vi "Steuerprogramm_ECD.vi"() -> ()   [LabVIEW 2017]
uses:
  <vilib>/FPGAPlugInAG/cRIO-9035/niLvFpga_Close_cRIO-9035.vi
  <vilib>/rvi/errors/niLvFpgaAdjustHostInterfaceError.vi
  <vilib>/Utility/error.llb/Error Cluster From Error Code.vi
  GVZeitenZyklen.vi
  GVHorstSP.vi
  gvbooleschRT.vi
  GVMethodenwechsel.vi
  GVaktuelleTDMS.vi
  GVChroms.vi
  GVMWHorst.vi
  GVVentilposition.vi
  GVMetavariablen.vi
  GVHK1Hz.vi
  GVZwangs.vi
  GVZwangsMPV.vi
  GVTrapsMachs.vi
  GVECDs.vi
  GVAIs.vi
  GVHeizenLH.vi
  GVProbenvol.vi
  <vilib>/rvi/interface/nirviCloseFPGA/nirviCloseFPGA.xnode
  FPGA Bitfiles/HAGAR-VECD_FPGATarget_FPGA-ProgrammECD_WS++LmW9gGg.lvbitx
  FPGA-Programm_ECD.vi
  <vilib>/rvi/interface/nirviReadWriteControl/nirviReadWriteControl.xnode
  <vilib>/rvi/interface/nirviMethod/nirviMethod.xnode
  <vilib>/rvi/errors/niLvFpgaMergeErrorWithErrorCode.vi
  <vilib>/FPGAPlugInAG/cRIO-9035/niLvFpga_WriteFifo_cRIO-9035.vi
  NiFpgaLv.dll
panel:
  in  "Methode speichern":bool
  out "ZyklusNummernGesamt":i32[](array[numeric])
  in  "veränderte Methode benutzen":bool
  in  "Methode verändern":bool
  out "ZyklusNummern":i32[](array[numeric])
  out "Big Ben, Methodenzeit, Zykluszeit0, Zykluszeit1, Zykluszeit2A, Zykluszeit2B":i32[](array[numeric])
  in  "global stop RT":bool
  in  "Methode":i32(ring) items=["Bedingsmethode", "Startmethode", "Meßmodus", "Shut-up-Methode", "Test", "HAG2 1/2", "Startmethode", "HAG2 1/2 Aufwärmen", "LicorDruckProfil1", "LicorDruckProfil2", "LicorDruckProfil0", "LicorDruckProfil3", "Kalibration-Meßmodus", "Kalibration-Meßmodus-II", "Kalibration-MesmodusIII", "Kalibration-Messmodus-IV", "Kalibration-ECD", "", "Kalibration-ECD-Blank"]
  in  "Registerkarte":T1(tab)
  out "SHOK?":bool[](array[boolean])
  out "schnelle Heizungen":string[](array[string])
  out "schnelle Heizungen":dbl[](array[numeric])
  out "HorstOK?":bool[](array[boolean])
  out "AIs3OK?":bool[](array[boolean])
  out "AIs1OK?":bool[](array[boolean])
  out "AIs1":dbl[](array[numeric])
  out "AIs1":string[](array[string])
  out "AIs2":string[](array[string])
  out "AIs3":string[](array[string])
  out "AIs2":dbl[](array[numeric])
  out "AIs3":dbl[](array[numeric])
  out "Metavariablen":string[](array[string])
  out "Metavariablen":dbl[](array[numeric])
  out "MWHorst":dbl[](array[numeric])
  out "HorstRegler":string[](array[string])
  out "AIs2OK?":bool[](array[boolean])
  out "Ventilposition":i32=1 min=1 max=6 step=1
  out "MVOK?":bool[](array[boolean])
  in  "LH-Gruppe":bool[](array[boolean])=[FALSE, FALSE, FALSE, FALSE, FALSE, FALSE, FALSE, FALSE, FALSE, FALSE, FALSE, FALSE]
  out "LangsameHeizungen":string[](array[string])
  out "Housekeeping1":cluster{dbl[], dbl[]}(graph)
  in  "Zeitachse1":i32(ring)=1 items=["Zykluszeit [s] Mod0", "Zykluszeit [s] Mod1", "Zykluszeit [s] Mod2A", "Zykluszeit [s] Mod2B"]
  in  "dargestellte Größe 1":i32(ring)=1 items=["T1-Spare1", "T1-Spare2", "T1-StirlingKühlkopf [°C]", "T1-PreCol1 [°C]", "T1-PreCol2 [°C]", "T1-MainCol1a [°C]", "T1-MainCol1b [°C]", "T1-MainCol2a [°C]", "T1-MainCol2b [°C]", "T1-BronkhorstUntena [°C]", "T1-BronkhorstUntenb [°C]", "T1-BronkhorstObena [°C]", "T1-BronkhorstObenb [°C]", "T1-2Pos1B [°C]", "T1-Spare9", "T1-2Pos1A [°C]", "T1-Spare10", "T1-TurboPump [°C]", "T1-StirlingPlatine [°C]", "T1-Spare5", "T1-Spare6", "T1-Spare7", "T1-Inlet [°C]", "F1-MFM-Spare", "F1-MFM0D [mL]", "P1-HeliumHP [bara]", "P1-HeliumLP [bara]", "P1-PumpVordruck [mbara]", "TurboSpeed", "I1-MS-AC [A]", "I1-Trap1 [A]", "I1-Trap2 [A]", "T2-ECD1a", "T2-ECD1b", "T2-ECD2a", "T2-ECD2b", "T2-Col1a", "T2-Col1b", "T2-Col2a", "T2-Col2b", "T2-Spare1", "T2-Spare2", "T2-Spare3", "T2-Spare4", "T2-Spare5", "T2-Spare6", "T2-Spare7", "F2-MFM2A", "F2-MFM2B", "F2-MFM2C", "P2-N2O_HP", "P2-N2O_LP", "P2-CO2_HP", "P2-CO2_LP", "AI-Spare1", "FL-MFM1000mL", "AI-Spare3", "AI-Spare4", "StirlingAlarm", "StirlingEmerg.", "AI-Spare7", "AI-Spare8", "AI-Spare9", "FL-MFM30mL", "T0-DC/DC5", "I0-24V_M0", "I0-48V_M1", "I0-24V_M1", "I0-28V_M2", "T0-Spare3", "T0-Spare2", "T0-Spare4", "T0-DC/DC7", "I0-20V_Laptop", "I0-28V_M1", "I0-24V_M2", "I0-12V_Licor", "T0-Spare1", "T0-Drier", "T0-Spare5", "F0-MFM0A [L]", "TL-Licor_a", "P0-Span-HP", "P0-spare1", "P0-Stickstoff-LP", "P0-Helium-LP", "P0-Cal-HP", "P0-P9Tavco[bar]", "F0-MFM0B [L]", "TL-Licor_b", "P0-Span-LP", "P0-spare2", "P0-Stickstoff-HP", "P0-Helium-HP", "P0-Cal-LP", "F0-MFM3", "TemperaturTrap1[°C]", "TemperaturTrap2[°C]", "TemperaturPreMach1[°C]", "TemperaturPreMach2[°C]", "TemperaturMainMach1[°C]", "TemperaturMainMach2[°C]", "PrC0 [bara]", "PrC0-Licor [bara]", "PrC1-Säule1 [bara]", "PrC1-Säule2 [bara]", "MFC1-Sample [ml/min]", "PrC1-BackFlush1 [bara]", "PrC1-BackFlush2 [bara]", "MFC1-Reaktant [l/min]", "MFC2A[ml/min]", "MFC2B[ml/min]", "MFC2C[ul/min]", "PrC2A[bara]", "MFC2D[ml/min]", "MFC2E[ml/min]", "PrC2B[bara]"]
  out "Housekeeping2":cluster{dbl[], dbl[]}(graph)
  in  "Zeitachse2":i32(ring)=1 items=["Zykluszeit [s] Mod0", "Zykluszeit [s] Mod1", "Zykluszeit [s] Mod2A", "Zykluszeit [s] Mod2B"]
  in  "dargestellte Größe 2":i32(ring)=1 items=["T1-Spare1", "T1-Spare2", "T1-StirlingKühlkopf [°C]", "T1-PreCol1 [°C]", "T1-PreCol2 [°C]", "T1-MainCol1a [°C]", "T1-MainCol1b [°C]", "T1-MainCol2a [°C]", "T1-MainCol2b [°C]", "T1-BronkhorstUntena [°C]", "T1-BronkhorstUntenb [°C]", "T1-BronkhorstObena [°C]", "T1-BronkhorstObenb [°C]", "T1-2Pos1B [°C]", "T1-Spare9", "T1-2Pos1A [°C]", "T1-Spare10", "T1-TurboPump [°C]", "T1-StirlingPlatine [°C]", "T1-Spare5", "T1-Spare6", "T1-Spare7", "T1-Inlet [°C]", "F1-MFM-Spare", "F1-MFM0D [mL]", "P1-HeliumHP [bara]", "P1-HeliumLP [bara]", "P1-PumpVordruck [mbara]", "TurboSpeed", "I1-MS-AC [A]", "I1-Trap1 [A]", "I1-Trap2 [A]", "T2-ECD1a", "T2-ECD1b", "T2-ECD2a", "T2-ECD2b", "T2-Col1a", "T2-Col1b", "T2-Col2a", "T2-Col2b", "T2-Spare1", "T2-Spare2", "T2-Spare3", "T2-Spare4", "T2-Spare5", "T2-Spare6", "T2-Spare7", "F2-MFM2A", "F2-MFM2B", "F2-MFM2C", "P2-N2O_HP", "P2-N2O_LP", "P2-CO2_HP", "P2-CO2_LP", "AI-Spare1", "FL-MFM1000mL", "AI-Spare3", "AI-Spare4", "StirlingAlarm", "StirlingEmerg.", "AI-Spare7", "AI-Spare8", "AI-Spare9", "FL-MFM30mL", "T0-DC/DC5", "I0-24V_M0", "I0-48V_M1", "I0-24V_M1", "I0-28V_M2", "T0-Spare3", "T0-Spare2", "T0-Spare4", "T0-DC/DC7", "I0-20V_Laptop", "I0-28V_M1", "I0-24V_M2", "I0-12V_Licor", "T0-Spare1", "T0-Drier", "T0-Spare5", "F0-MFM0A [L]", "TL-Licor_a", "P0-Span-HP", "P0-spare1", "P0-Stickstoff-LP", "P0-Helium-LP", "P0-Cal-HP", "P0-P9Tavco[bar]", "F0-MFM0B [L]", "TL-Licor_b", "P0-Span-LP", "P0-spare2", "P0-Stickstoff-HP", "P0-Helium-HP", "P0-Cal-LP", "F0-MFM3", "TemperaturTrap1[°C]", "TemperaturTrap2[°C]", "TemperaturPreMach1[°C]", "TemperaturPreMach2[°C]", "TemperaturMainMach1[°C]", "TemperaturMainMach2[°C]", "PrC0 [bara]", "PrC0-Licor [bara]", "PrC1-Säule1 [bara]", "PrC1-Säule2 [bara]", "MFC1-Sample [ml/min]", "PrC1-BackFlush1 [bara]", "PrC1-BackFlush2 [bara]", "MFC1-Reaktant [l/min]", "MFC2A[ml/min]", "MFC2B[ml/min]", "MFC2C[ul/min]", "PrC2A[bara]", "MFC2D[ml/min]", "MFC2E[ml/min]", "PrC2B[bara]"]
  out "Detektor 2":cluster{dbl[], dbl[]}[](graph)
  in  "Detektor":i32(ring) items=["ECD1", "ECD2"]
  in  "HK1YMin":dbl
  in  "HK1YMax":dbl=100.0
  in  "HK2YMin":dbl
  in  "HK2YMax":dbl=100.0
  in  "DetYMin":dbl
  in  "DetYMax":dbl=100.0
  in  "NeuerRefstrom":bool
  in  "RefStromECD1":i16 min=0 max=2500 step=1
  in  "RefStromECD2":i16 min=0 max=2500 step=1
  out "schnelleAnzeige":cluster{dbl[], dbl[]}(graph)
  in  "TafelWischen!":bool
  in  "dargestellte Größe 3":i32(ring)=1 items=["TemperaturTrap1[°C]", "TemperaturTrap2[°C]", "TemperaturPreMach1[°C]", "TemperaturPreMach2[°C]", "TemperaturMainMach1[°C]", "TemperaturMainMach2[°C]", "PrC0 [bara]", "PrC0-Licor [bara]", "PrC1-Säule1 [bara]", "PrC1-Säule2 [bara]", "MFC1-Sample [ml/min]", "PrC1-BackFlush1 [bara]", "PrC1-BackFlush2 [bara]", "MFC1-Reaktant [l/min]", "MFC2A[ml/min]", "MFC2B[ml/min]", "MFC2C[ul/min]", "PrC2A[bara]", "MFC2D[ml/min]", "MFC2E[ml/min]", "PrC2B[bara]"]
  in  "An/Aus":bool
  out "TDMSwriteECD":errorcluster
  out "AIsFIFOread":errorcluster
  out "MWTrapsMachs":errorcluster
  out "TDMSwriteHK":errorcluster
  out "TDMScloseHK":errorcluster
  out "TDMSopenHK":errorcluster
  out "TDMScloseECD2":errorcluster
  out "TDMSopenECD2":errorcluster
  out "TDMScloseECD1":errorcluster
  out "TDMSopenECD1":errorcluster
  out "FIFOwriteRS485":errorcluster
  out "SerielleKomm.":errorcluster
  out "LH":errorcluster
  out "Zyklus":errorcluster
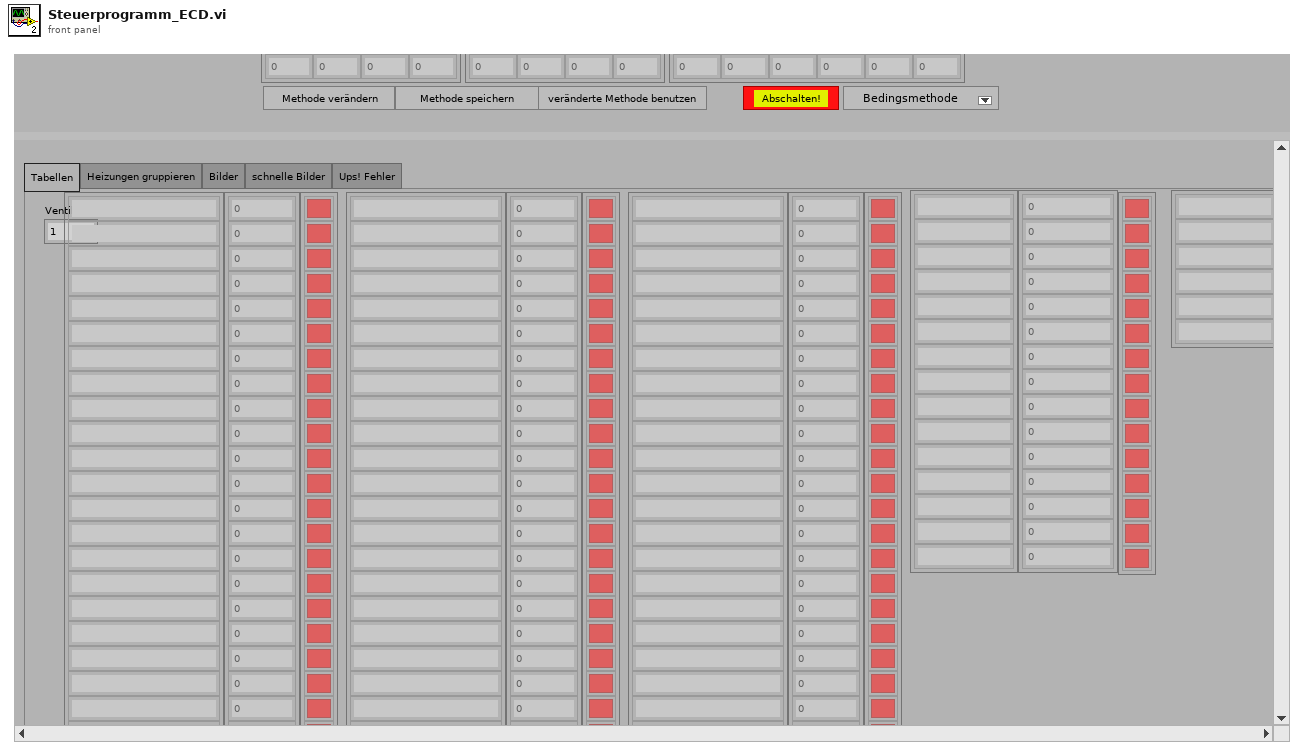
[diagram p1: front panel]
types:
  T1 = enum32{"Tabellen", "Heizungen gruppieren", "Bilder", "schnelle Bilder", "Ups! Fehler"}
  T2 = cluster{"DIOsMod0Nr":i32[], "DIOsMod1Nr":i32[], "DIOsMod2ANr":i32[], "DIOsMod2BNr":i32[], "AIsLH":i32[], "AnzahlRegler/Modul":i32[], "Regler für den Probenfluß":i32, "SPvorgebenMod0":string[], "SPvorgebenMod1":string[], "SPvorgebenMod2A":string[], "SPvorgebenMod2B":string[], "MWAntwortMod0":string[], "MWAntwortMod1":string[], "MWAntwortMod2A":string[], "MWAntwortMod2B":string[], "FaktorMod0":dbl[], "FaktorMod1":dbl[], "FaktorMod2A":dbl[], "FaktorMod2B":dbl[], "MWabfragenMod0":string[], "MWabfragenMod1":string[], "MWabfragenMod2A":string[], "MWabfragenMod2B":string[], "Modul1/AI koeff":dbl[][], "Modul2/AI koeff":dbl[][], "Modul3/AI koeff":dbl[][], "Traps/MachsKoeff T(R)":dbl[][], "Modul1/AIsNamen":string[], "Modul2/AIsNamen":string[], "Modul3/AIsNamen":string[], "DIOsMod0Name":string[], "DIOsMod1Name":string[], "DIOsMod2AName":string[], "DIOsMod2BName":string[], "ReglerNameMod0":string[], "ReglerNameMod1":string[], "ReglerNameMod2A":string[], "ReglerNameMod2B":string[], "Startmethode":i32, "Dateiordner Housekeeping":path, "Dateiname Housekeeping":string, "DateiordnerECD1":path, "DateinameECD1":string, "DateiordnerECD2":path, "DateinameECD2":string, "LangsameHeizungen":string[], "ModuleLH":i32[], "Metavariablen":string[], "Modul1/AI sicherer Bereich":dbl[][], "Modul2/AI sicherer Bereich":dbl[][], "Modul3/AI sicherer Bereich":dbl[][], "Traps/Machs sicherer Bereich":dbl[][], "ReglerMod0 sicherer Bereich":dbl[][], "ReglerMod1 sicherer Bereich":dbl[][], "ReglerMod2A sicherer Bereich":dbl[][], "ReglerMod2B sicherer Bereich":dbl[][], "Metavariablen grüner Bereich":dbl[][], "Traps/MachsKoeff R(U)":dbl[][], "LHGruppe":bool[]}
  T3 = cluster{"Zykluslängen [s]":dbl[], "ZeitpktDIOsMod0":dbl[], "ZeitpktDIOsMod1":dbl[], "ZeitpktDIOsMod2A":dbl[], "ZeitpktDIOsMod2B":dbl[], "DIOsSPMod0":bool[][], "DIOsSPMod1":bool[][], "DIOsSPMod2A":bool[][], "DIOsSPMod2B":bool[][], "Mod0HorstZeitpkt":dbl[], "Mod1HorstZeitpkt":dbl[], "Mod2AHorstZeitpkt":dbl[], "Mod2BHorstZeitpkt":dbl[], "HorstSPMod0":dbl[][], "HorstSPMod1":dbl[][], "HorstSPMod2A":dbl[][], "HorstSPMod2B":dbl[][], "LHSetpoints":dbl[], "LHHeizen?":bool[], "ZPktFPGABoolesch":dbl[], "FPGABoolesch":bool[][], "ZeitpktFPGAPID":dbl[], "FPGAPID":cluster{"d0":fxp<+/-,18,18>, "d1":fxp<+/-,21,21>}[][], "ZeitpktFPGAFixp":dbl[], dbl[][], "t_PreMach1":dbl[], "T_PreMach1":dbl[], "t_PreMach2":dbl[], "T_PreMach2":dbl[], "PIDs für \"träge\" Heizungen":cluster{"proportional gain (Kc)":dbl, "integral time (Ti, min)":dbl, "derivative time (Td, min)":dbl}[], "Zwangsbedingungen":dbl[][], "Dateien fürs MS schicken?":bool, "ZeitpunkteMPV":dbl[], "SPMPV":i32[], "ZeitpktMS-1":dbl, "ZeitpktMS-2":dbl, "Int.Start1":dbl, "Int.Stop1":dbl, "Int.Start2":dbl, "Int.Stop2":dbl, "Methodenname":string, "t_MainMach1":dbl[], "T_MainMach1":dbl[], "t_MainMach2":dbl[], "T_MainMach2":dbl[]}[]
  T4 = enum16{"open", "replace", "create", "open or create", "replace or create", "replace or create with confirmation"}
  T5 = cluster{"Zyklus1":i32, "Zeitachse1":i32, "dargestellte Größe 1":i32, "Zyklus2":i32, "Zeitachse2":i32, "dargestellte Größe 2":i32}
  T6 = cluster{"DIOsMod0Name":string[], "DIOsMod1Name":string[], "DIOsMod2AName":string[], "DIOsMod2BName":string[], "ReglerNameMod0":string[], "ReglerNameMod1":string[], "ReglerNameMod2A":string[], "ReglerNameMod2B":string[], "LangsameHeizungen":string[]}
  T7 = cluster{"Zykluslängen [s]":dbl[], "ZeitpktDIOsMod0":dbl[], "ZeitpktDIOsMod1":dbl[], "ZeitpktDIOsMod2A":dbl[], "ZeitpktDIOsMod2B":dbl[], "DIOsSPMod0":bool[][], "DIOsSPMod1":bool[][], "DIOsSPMod2A":bool[][], "DIOsSPMod2B":bool[][], "Mod0HorstZeitpkt":dbl[], "Mod1HorstZeitpkt":dbl[], "Mod2AHorstZeitpkt":dbl[], "Mod2BHorstZeitpkt":dbl[], "HorstSPMod0":dbl[][], "HorstSPMod1":dbl[][], "HorstSPMod2A":dbl[][], "HorstSPMod2B":dbl[][], "LHSetpoints":dbl[], "LHHeizen?":bool[], "ZPktFPGABoolesch":dbl[], "FPGABoolesch":bool[][], "ZeitpktFPGAPID":dbl[], "FPGAPID":cluster{"d0":fxp<+/-,18,18>, "d1":fxp<+/-,21,21>}[][], "ZeitpktFPGAFixp":dbl[], dbl[][], "t_PreMach1":dbl[], "T_PreMach1":dbl[], "t_PreMach2":dbl[], "T_PreMach2":dbl[], "PIDs für \"träge\" Heizungen":cluster{"proportional gain (Kc)":dbl, "integral time (Ti, min)":dbl, "derivative time (Td, min)":dbl}[], "Zwangsbedingungen":dbl[][], "Dateien fürs MS schicken?":bool, "ZeitpunkteMPV":dbl[], "SPMPV":i32[], "ZeitpktMS-1":dbl, "ZeitpktMS-2":dbl, "Int.Start1":dbl, "Int.Stop1":dbl, "Int.Start2":dbl, "Int.Stop2":dbl, "Methodenname":string, "t_MainMach1":dbl[], "T_MainMach1":dbl[], "t_MainMach2":dbl[], "T_MainMach2":dbl[]}
  T8 = cluster{"Modul1/AI sicherer Bereich":dbl[][], "Modul2/AI sicherer Bereich":dbl[][], "Modul3/AI sicherer Bereich":dbl[][], "Traps/Machs sicherer Bereich":dbl[][], dbl[][], "Metavariablen grüner Bereich":dbl[][]}
  T9 = cluster{"created path":path, "created path":path, "created path":path, "Dateiname Housekeeping":string, "DateinameECD1":string, "DateinameECD2":string, "tdms0":refnum<k34>, "tdms1":refnum<k34>, "tdms0":refnum<k34>, "tdms1":refnum<k34>, "tdms0":refnum<k34>, "tdms1":refnum<k34>}
  T10 = cluster{"d0":fxp<+/-,18,18>, "d1":fxp<+/-,21,21>}[][]
  T11 = cluster{"proportional gain (Kc)":dbl, "integral time (Ti, min)":dbl, "derivative time (Td, min)":dbl}[]
  T12 = cluster{cluster{"ZeitpktDIOsMod2B":dbl[]}[], cluster{"DIOsSPMod2B":bool[][]}[], cluster{"Mod2BHorstZeitpkt":dbl[]}[], cluster{"HorstSPMod2B":dbl[][]}[], "LHHeizen?":bool[], "ZPktFPGABoolesch":dbl[], "FPGABoolesch":bool[][], "ZeitpktFPGAPID":dbl[], "FPGAPID":cluster{"d0":fxp<+/-,18,18>, "d1":fxp<+/-,21,21>}[][], "ZeitpktFPGAFixp":dbl[], dbl[][], "t_PreMach1":dbl[], "T_PreMach1":dbl[], "t_PreMach2":dbl[], "T_PreMach2":dbl[], "ZeitpunkteMPV":dbl[], "SPMPV":i32[], "t_MainMach1":dbl[], "T_MainMach1":dbl[], "t_MainMach2":dbl[], "T_MainMach2":dbl[]}
  T13 = cluster{"Zykluslängen [s]":dbl[], "ZeitpktDIOsMod0":dbl[], "ZeitpktDIOsMod1":dbl[], "ZeitpktDIOsMod2A":dbl[], "ZeitpktDIOsMod2B":dbl[], "DIOsSPMod0":bool[][], "DIOsSPMod1":bool[][], "DIOsSPMod2A":bool[][], "DIOsSPMod2B":bool[][], "Mod0HorstZeitpkt":dbl[], "Mod1HorstZeitpkt":dbl[], "Mod2AHorstZeitpkt":dbl[], "Mod2BHorstZeitpkt":dbl[], "HorstSPMod0":dbl[][], "HorstSPMod1":dbl[][], "HorstSPMod2A":dbl[][], "HorstSPMod2B":dbl[][], "LangsameHeizungenSP":dbl[], "LHHeizen?":bool[], "ZPktFPGABoolesch":dbl[], "FPGABoolesch":bool[][], "ZeitpktFPGAPID":dbl[], "FPGAPID":cluster{"d0":fxp<+/-,18,18>, "d1":fxp<+/-,21,21>}[][], "ZeitpktFPGAFixp":dbl[], "FPGAFixp":dbl[][], "t_PreMach1":dbl[], "T_PreMach1":dbl[], "t_PreMach2":dbl[], "T_PreMach2":dbl[], "PIDs für \"träge\" Heizungen":cluster{"proportional gain (Kc)":dbl, "integral time (Ti, min)":dbl, "derivative time (Td, min)":dbl}[], "Zwangsbedingungen":dbl[][], "MS-Daten?":bool, "ZeitpunkteMPV":dbl[], "SetpointMPV":i32[], "ZeitpktMS-1":dbl, "ZeitpktMS-2":dbl, "Int.Start1":dbl, "Int.Stop1":dbl, "Int.Start2":dbl, "Int.Stop2":dbl, "Methodenname":string, "t_MainMach1":dbl[], "T_MainMach1":dbl[], "t_MainMach2":dbl[], "T_MainMach2":dbl[]}
  T14 = cluster{"ZyklusNummern":i32[], "ZeilennummernDIOs":i32[], "ZwangsDIO?":cluster{bool[]}[], "ZeilennummernHorst":i32[], "ZwangsHorst?":cluster{bool[]}[], "ZeileFPGABoolesch":i32, "ZwangsFPGABoolesch?":bool[], "ZeileFPGAPID":i32, "ZeileFPGAFixp":i32, "ZeilePreMach1":i32, "ZeilePreMach2":i32, "ZeilennummerMPV":i32, "ZeileMainMach1":i32, "ZeileMainMach2":i32, "ZwangsMPV?":bool}
  T15 = cluster{"ZyklusNummern":i32[], i32[], "ZwangsDIO?":cluster{bool[]}[], i32[], "ZwangsHorst?":cluster{bool[]}[], i32, "ZwangsFPGABoolesch?":bool[], i32, i32, "ZeileMach":i32, "ZeileMach":i32, i32, "ZeileMach":i32, "ZeileMach":i32, "ZwangsMPV?":bool}
  T16 = cluster{string[], string[], string[], dbl[], dbl[], dbl[]}
  T17 = cluster{"Befehle1":string[], "Befehle2":string[], "Befehle3":string[]}
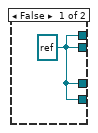
[diagram p2: hidden frame]
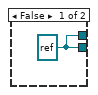
[diagram p3: hidden frame]
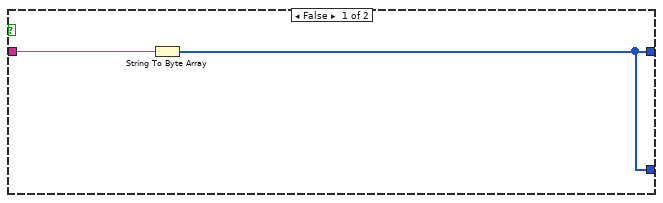
[diagram p6: hidden frame]
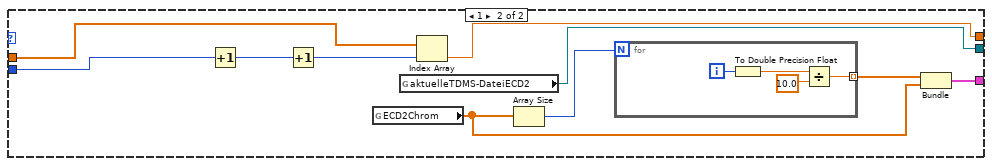
[diagram p13: hidden frame]
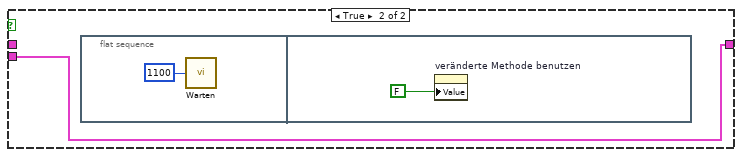
[diagram p14: hidden frame]
diagram:
  n1 = Open/Create/Replace File(file path (use dialog)=path "c:/einstellungen.pery" ("Datei (Dialog verwenden)"), operation (0:open)=T4."open" ("Operation (0:Öffnen)")) -> (refnum out=w13:refnum<file>)  [unwired: 4 in, 2 out]
  n2 = Open/Create/Replace File(file path (use dialog)=path "c:/methoden.pery" ("Datei (Dialog verwenden)"), operation (0:open)=T4."open" ("Operation (0:Öffnen)")) -> (refnum out=w8:refnum<file>)  [unwired: 4 in, 2 out]
  n3 = Read from Binary File(5:T2 {"DIOsMod0Nr"=[], "DIOsMod1Nr"=[], "DIOsMod2ANr"=[], "DIOsMod2BNr"=[], "AIsLH"=[], "AnzahlRegler/Modul"=[], "Regler für den Probenfluß"=0, "SPvorgebenMod0"=[], "SPvorgebenMod1"=[], "SPvorgebenMod2A"=[], "SPvorgebenMod2B"=[], "MWAntwortMod0"=[], "MWAntwortMod1"=[], "MWAntwortMod2A"=[], "MWAntwortMod2B"=[], "FaktorMod0"=[], "FaktorMod1"=[], "FaktorMod2A"=[], "FaktorMod2B"=[], "MWabfragenMod0"=[], "MWabfragenMod1"=[], "MWabfragenMod2A"=[], "MWabfragenMod2B"=[], "Modul1/AI koeff"=[], "Modul2/AI koeff"=[], "Modul3/AI koeff"=[], "Traps/MachsKoeff T(R)"=[], "Modul1/AIsNamen"=[], "Modul2/AIsNamen"=[], "Modul3/AIsNamen"=[], "DIOsMod0Name"=[], "DIOsMod1Name"=[], "DIOsMod2AName"=[], "DIOsMod2BName"=[], "ReglerNameMod0"=[], "ReglerNameMod1"=[], "ReglerNameMod2A"=[], "ReglerNameMod2B"=[], "Startmethode"=0, "Dateiordner Housekeeping"=path "", "Dateiname Housekeeping"="", "DateiordnerECD1"=path "", "DateinameECD1"="", "DateiordnerECD2"=path "", "DateinameECD2"="", "LangsameHeizungen"=[], "ModuleLH"=[], "Metavariablen"=[], "Modul1/AI sicherer Bereich"=[], "Modul2/AI sicherer Bereich"=[], "Modul3/AI sicherer Bereich"=[], "Traps/Machs sicherer Bereich"=[], "ReglerMod0 sicherer Bereich"=[], "ReglerMod1 sicherer Bereich"=[], "ReglerMod2A sicherer Bereich"=[], "ReglerMod2B sicherer Bereich"=[], "Metavariablen grüner Bereich"=[], "Traps/MachsKoeff R(U)"=[], "LHGruppe"=[]} ("Ausgangs-Cluster"), 11:w13) -> (2:w11:T2, 3:w12:refnum<file>)  [unwired: 4 in, 2 out]
  n4 = Read from Binary File(5:T3 [], 11:w8) -> (2:w6:T3, 3:w7:refnum<file>)  [unwired: 4 in, 2 out]
  n5 = Close File(refnum=w12) -> ()  [unwired: 1 in, 2 out]
  n6 = Close File(refnum=w7) -> ()  [unwired: 1 in, 2 out]
  n7 = flat-sequence {
    tunnel: [w44] -> w41
    tunnel: [w114] -> w40
    tunnel: [w48] -> w38
    tunnel: [w247] -> w37
    tunnel: [w249] -> w36
    tunnel: [w241] -> w35
    tunnel: [w248] -> w34
    tunnel: [w171] -> w33
    tunnel: [w240] -> w32
    tunnel: [w239] -> w31
    tunnel: [w233] -> w30
    tunnel: [w174] -> w29
    tunnel: [w148] -> w28
    tunnel: [w246] -> w27
    tunnel: [w238] -> w26
    tunnel: [w237] -> w25
    tunnel: [w229] -> w24
    tunnel: [w228] -> w23
    tunnel: [w227] -> w22
    tunnel: [w226] -> w21
    tunnel: [w225] -> w20
    tunnel: [w224] -> w19
    tunnel: [w221] -> w18
    tunnel: [w203] -> w17
    tunnel: w11 -> [w90]
    tunnel: [w202] -> w16
    tunnel: w6 -> [w115]
    tunnel: [w114] -> w5
    tunnel: [w90] -> w4
    tunnel: [w57] -> w3
    tunnel: w41 -> [w316]
    tunnel: w40 -> [w387]
    tunnel: [w316] -> w39
    tunnel: w38 -> [_]
    tunnel: w37 -> [w346]
    tunnel: w36 -> [w283]
    tunnel: w35 -> [w347]
    tunnel: w34 -> [w345]
    tunnel: w33 -> [w320]
    tunnel: w32 -> [w315]
    tunnel: w31 -> [w312]
    tunnel: w30 -> [w309]
    tunnel: w29 -> [w310]
    tunnel: w28 -> [w313]
    tunnel: w27 -> [w385]
    tunnel: w26 -> [w318]
    tunnel: w25 -> [w386]
    tunnel: w24 -> [w291]
    tunnel: w23 -> [w290]
    tunnel: w22 -> [w289]
    tunnel: w21 -> [w383]
    tunnel: w20 -> [w382]
    tunnel: w19 -> [w381]
    tunnel: w18 -> [w337]
    tunnel: w17 -> [w319]
    tunnel: w16 -> [w308]
    tunnel: w6 -> [w307]
    tunnel: w5 -> [w305]
    tunnel: w4 -> [_]
    tunnel: w3 -> [w284]
    tunnel: w39 -> [w1070]
    frame #0 {
      w116 = TRUE
      w130 = 0.0 ("Probenvol.1")
      w137 = dbl[] [-1.0] ("ECD1MW")
      w138 = FALSE ("ECD1Empfangen?")
      w129 = string[] ["TemperaturTrap1[°C]", "TemperaturTrap2[°C]", "TemperaturPreMach1[°C]", "TemperaturPreMach2[°C]", "TemperaturMainMach1[°C]", "TemperaturMainMach2[°C]"]
      w244 = string[] ["Big Ben [s]", "Methodenzeit [s]", "Zykluszeit [s] Mod0", "Zykluszeit [s] Mod1", "Zykluszeit [s] Mod2A", "Zykluszeit [s] Mod2B"]
      w234 = FALSE ("Undefinierte Werte möglich")
      w235 = FALSE ("global stop RT")
      n8 = for {
        tunnel: [w277] -> w242 mode=indexing
        tunnel: w115 -> [w278] mode=indexing
        n9 = Unbundle(w278) -> ("Methodenname"=w277:string)  [unwired: 44 out]
      }
      n10 = Unbundle(w90) -> ("DIOsMod0Nr"=w158:i32[], "DIOsMod1Nr"=w157:i32[], "DIOsMod2ANr"=w156:i32[], "DIOsMod2BNr"=w155:i32[], "AIsLH"=w145:i32[], "AnzahlRegler/Modul"=w148:i32[], "Regler für den Probenfluß"=w202:i32, "SPvorgebenMod0"=w201:string[], "SPvorgebenMod1"=w200:string[], "SPvorgebenMod2A"=w199:string[], "SPvorgebenMod2B"=w198:string[], "MWAntwortMod0"=w197:string[], "MWAntwortMod1"=w196:string[], "MWAntwortMod2A"=w195:string[], "MWAntwortMod2B"=w194:string[], "FaktorMod0"=w193:dbl[], "FaktorMod1"=w192:dbl[], "FaktorMod2A"=w191:dbl[], "FaktorMod2B"=w190:dbl[], "MWabfragenMod0"=w189:string[], "MWabfragenMod1"=w188:string[], "MWabfragenMod2A"=w187:string[], "MWabfragenMod2B"=w186:string[], "Modul1/AI koeff"=w185:dbl[][], "Modul2/AI koeff"=w184:dbl[][], "Modul3/AI koeff"=w183:dbl[][], "Traps/MachsKoeff T(R)"=w182:dbl[][], "Modul1/AIsNamen"=w181:string[], "Modul2/AIsNamen"=w180:string[], "Modul3/AIsNamen"=w179:string[], "DIOsMod0Name"=w88:string[], "DIOsMod1Name"=w89:string[], "DIOsMod2AName"=w87:string[], "DIOsMod2BName"=w86:string[], "ReglerNameMod0"=w105:string[], "ReglerNameMod1"=w104:string[], "ReglerNameMod2A"=w103:string[], "ReglerNameMod2B"=w102:string[], "Startmethode"=w114:i32, "Dateiordner Housekeeping"=w85:path, "Dateiname Housekeeping"=w178:string, "DateiordnerECD1"=w99:path, "DateinameECD1"=w177:string, "DateiordnerECD2"=w98:path, "DateinameECD2"=w176:string, "LangsameHeizungen"=w175:string[], "ModuleLH"=w170:i32[], "Metavariablen"=w109:string[], "Modul1/AI sicherer Bereich"=w61:dbl[][], "Modul2/AI sicherer Bereich"=w60:dbl[][], "Modul3/AI sicherer Bereich"=w59:dbl[][], "Traps/Machs sicherer Bereich"=w58:dbl[][], "ReglerMod0 sicherer Bereich"=w56:dbl[][], "ReglerMod1 sicherer Bereich"=w55:dbl[][], "ReglerMod2A sicherer Bereich"=w54:dbl[][], "ReglerMod2B sicherer Bereich"=w53:dbl[][], "Metavariablen grüner Bereich"=w51:dbl[][], "LHGruppe"=w43:bool[])  [unwired: 1 out]
      "Metavariablen" <- w109
      "LangsameHeizungen" <- w175
      n11 = Initialize Array(0, 4 ("Dimension")) -> (w131:i32[])
      n12 = Initialize Array(0.0 ("Element"), 6 ("Dimension")) -> (w134:dbl[])
      n13 = global write "GVMethodenwechsel.vi" "Methodenwechsel?"(FALSE ("Methodenwechsel?")) -> ()
      n14 = local write "NeuerRefstrom"(FALSE ("NeuerRefstrom")) -> ()
      n15 = property on="dargestellte Größe 2" class="Ring (strikt)"("AllowUndefVals"=w234) -> ()  [unwired: 2 in, 2 out]
      n16 = property on="Zeitachse2" class="Ring (strikt)"("AllowUndefVals"=w234) -> ()  [unwired: 2 in, 2 out]
      n17 = property on="Zeitachse1" class="Ring (strikt)"("AllowUndefVals"=w234) -> ()  [unwired: 2 in, 2 out]
      n18 = property on="dargestellte Größe 1" class="Ring (strikt)"("AllowUndefVals"=w234) -> ()  [unwired: 2 in, 2 out]
      n19 = property on="Methode" class="Ring (strikt)"("AllowUndefVals"=w234) -> ()  [unwired: 2 in, 2 out]
      n20 = global write "GVProbenvol.vi" "Probenvol.1"(w130) -> ()
      n21 = global write "GVProbenvol.vi" "Probenvol.2"(w130) -> ()
      n22 = global write "GVECDs.vi" "ECD1MW"(w137) -> ()
      n23 = global write "GVECDs.vi" "ECD2MW"(w137) -> ()
      n24 = global write "GVECDs.vi" "ECD1Empfangen?"(w138) -> ()
      n25 = global write "GVECDs.vi" "ECD2Empfangen?"(w138) -> ()
      n26 = local write "global stop RT"(w235) -> ()
      n27 = global write "gvbooleschRT.vi" "global stop RT"(w235) -> ()
      n28 = global write "GVZeitenZyklen.vi" "ZyklusNummern"(w131) -> ()
      n29 = global write "GVZeitenZyklen.vi" "ZyklusNummernGesamt"(w131) -> ()
      n30 = global write "GVZeitenZyklen.vi" "Big Ben, Methodenzeit, Zykluszeit0, Zykluszeit1, Zykluszeit2A, Zykluszeit2B"(w134) -> ()
      n31 = property on="Methode" class="Ring (strikt)"("Value"=w114) -> ()  [unwired: 2 in, 2 out]
      n32 = Initialize Array(-1.0 ("Element"), 6 ("Dimension")) -> (w141:dbl[])
      n33 = Initialize Array(FALSE, 10 ("Dimension")) -> (w149:bool[])
      n34 = Initialize Array(-1.0 ("Element"), 96 ("Dimension")) -> (w142:dbl[])
      n35 = local write "LH-Gruppe"(w43) -> ()
      n36 = global write "GVZwangs.vi" "ZwangsFPGABoolesch!"(w149) -> ()
      n37 = global write "GVZwangs.vi" "ZwangsFPGABoolesch?"(w149) -> ()
      n38 = global write "GVTrapsMachs.vi" "Traps/Machs"(w141) -> ()
      n39 = global write "GVAIs.vi" "AIs"(w142) -> ()
      n40 = for {
        tunnel: w148 -> [w255] mode=indexing
        tunnel: [w252] -> w147 mode=indexing
        tunnel: [w250] -> w146 mode=indexing
        n41 = Initialize Array(0.0 ("Element"), w255) -> (w253:dbl[])
        n42 = Initialize Array(FALSE, w255) -> (w251:bool[])
        n43 = Bundle(w253) -> (w252:cluster{dbl[]})  [unwired: 1 in]
        n44 = Bundle(w251) -> (w250:cluster{bool[]})  [unwired: 1 in]
      }
      n45 = Bundle("DIOsMod0Name"=w88, "DIOsMod1Name"=w89, "DIOsMod2AName"=w87, "DIOsMod2BName"=w86, "ReglerNameMod0"=w105, "ReglerNameMod1"=w104, "ReglerNameMod2A"=w103, "ReglerNameMod2B"=w102, "LangsameHeizungen"=w175) -> (w237:T6)  [unwired: 1 in]
      n46 = Build Array (concatenate)(w105, w104, w103, w102) -> (w128:string[])
      n47 = Build Array (concatenate)(w197, w196, w195, w194) -> (w248:string[])
      n48 = Build Array (concatenate)(w201, w200, w199, w198) -> (w249:string[])
      n49 = Build Array (concatenate)(w193, w192, w191, w190) -> (w241:dbl[])
      n50 = Build Array (concatenate)(w189, w188, w187, w186) -> (w247:string[])
      n51 = Build Array (concatenate)(w105, w104, w103, w102) -> (→"HorstRegler":string[])
      n52 = Build Array (concatenate)(w56, w55, w54, w53) -> (w52:dbl[][])
      n53 = Array Size(array=w109) -> (size(s)=w108:i32)
      n54 = Build Array(w158, w157, w156, w155) -> (w154:i32[][])
      n55 = Array Size(array=w175) -> (size(s)=w174:i32)
      n56 = Add Array Elements(numeric array=w148) -> (sum=w233:i32)
      n57 = Array Size(array=w145) -> (size(s)=w144:i32)
      n58 = Index Array(array=w115, index=w114) -> (element=w113:T7)
      n59 = Add Array Elements(numeric array=w148) -> (sum=w160:i32)
      n60 = Decrement(x=w170) -> (x-1=w169:i32[])
      n61 = Build Cluster Array(w158, w157, w156, w155) -> (w240:cluster{"DIOsMod2BNr":i32[]}[])
      n62 = Build Array (concatenate)(w181, w180, w179) -> (w42:string[])
      n63 = Index Array(array=w182, index (col)=2 ("Deaktivierter Index (Spalte)")) -> (element=w229:dbl[])  [unwired: 1 in]
      n64 = Index Array(array=w182, index (col)=0 ("Deaktivierter Index (Spalte)")) -> (element=w227:dbl[])  [unwired: 1 in]
      n65 = Index Array(array=w182, index (col)=1 ("Deaktivierter Index (Spalte)")) -> (element=w228:dbl[])  [unwired: 1 in]
      n66 = Concatenate Strings("?SE0,SETP,1700" ("string"), "\n") -> (w63:string)
      n67 = Concatenate Strings("?SE0,SETP,2200" ("string"), "\n") -> (w70:string)
      n68 = for {
        tunnel: w240 -> [w280] mode=indexing
        tunnel: [w281] -> w239 mode=indexing
        n69 = Unbundle(w280) -> ("DIOsMod2BNr"=w279:i32[])
        n70 = Array Size(array=w279) -> (size(s)=w281:i32)
      }
      n71 = property on="Methode" class="Ring (strikt)"("Strings []"=w242) -> ()  [unwired: 2 in, 2 out]
      n72 = Bundle("Modul1/AI sicherer Bereich"=w61, "Modul2/AI sicherer Bereich"=w60, "Modul3/AI sicherer Bereich"=w59, "Traps/Machs sicherer Bereich"=w58, w52, "Metavariablen grüner Bereich"=w51) -> (w57:T8)  [unwired: 1 in]
      n73 = Build Array (concatenate)(w142, w141) -> (w140:dbl[])
      n74 = Array Size(array=w154) -> (size(s)=w153:i32[])
      n75 = Unbundle(w113) -> ("SPMPV"=w112:i32[])  [unwired: 44 out]
      n76 = Open/Create/Replace File(file path (use dialog)=path "c:/fromcriordy.txt" ("Dateipfad (Dialog verwenden)"), operation (0:open)=T4."replace or create" ("Operation (0:Öffnen)")) -> (refnum out=w206:refnum<file>, error out=w207:errorcluster)  [unwired: 4 in, 1 out]
      n77 = Initialize Array(0.0 ("element"), w108) -> (w106:dbl[])
      n78 = Initialize Array(0.0 ("Element"), w160) -> (w159:dbl[])
      n79 = Get Date/Time In Seconds() -> (seconds since 1Jan1904=w100:timestamp)
      n80 = Initialize Array(FALSE, w144) -> (w139:bool[])
      n81 = Multiply(x=w169, y=32) -> (x*y=w172:i32[])
      n82 = Initialize Array(-1.0, w160) -> (w162:dbl[])
      n83 = Array Subset(array=w42, index=32 ("Index"), length=32 ("Länge")) -> (→"AIs2":string[])
      n84 = Array Subset(array=w42, index=0 ("Index"), length=32 ("Länge")) -> (→"AIs1":string[])
      n85 = Array Subset(array=w42, index=64 ("Index"), length=32 ("Länge")) -> (→"AIs3":string[])
      n86 = global write "GVHK1Hz.vi" "Mod1Mod2Mod3/AITrapsMachs1Hz"(w140) -> ()
      n87 = global write "GVMetavariablen.vi" "Metavariablen"(w106) -> ()
      n88 = global write "GVHeizenLH.vi" "Heizen?LH"(w139) -> ()
      n89 = global write "GVZwangs.vi" "ZwangsLangsameHeizungenAn!"(w139) -> ()
      n90 = for {
        tunnel: w153 -> [w260] mode=indexing
        tunnel: [w257] -> w152 mode=indexing
        n91 = Initialize Array(FALSE, w260) -> (w258:bool[])
        n92 = Bundle(w258) -> (w257:cluster{bool[]})  [unwired: 1 in]
      }
      n93 = global write "GVHorstSP.vi" "HorstSP"(w159) -> ()
      n94 = global write "GVZwangs.vi" "ZwangsLangsameHeizungenAn?"(w139) -> ()
      n95 = Add(x=w172, y=w145) -> (x+y=w171:i32[])
      n96 = Close File(refnum=w206, error in=w207) -> (path=w238:path)  [unwired: 1 out]
      n97 = Format Date/Time String(time format string (%c)="%Y-%m-%d--%H-%M" ("Zeitformatierungs-String (%c)"), seconds (now)=w100) -> (date/time string=w78:string)  [unwired: 1 in]
      n98 = String To Byte Array(string=w63) -> (unsigned byte array=w65:u8[])
      n99 = String To Byte Array(string=w70) -> (unsigned byte array=w75:u8[])
      n100 = Index Array(array=w112, index=0) -> (element=w110:i32)
      n101 = call "FPGA-Start_ECD.vi"() -> ("error out"=w48:errorcluster, "FPGA-VI-Referenz (Ausgang)"=w47:refnum<k20>)  [unwired: 2 in]
      n102 = global write "GVMWHorst.vi" "MWHorst"(w162) -> ()
      n103 = global write "GVVentilposition.vi" "Ventilposition"(w110) -> ()
      n104 = Build Array (concatenate)(string[] ["Jahr", "Monat", "Tag", "Stunde", "Minute", "Sekunde"] ("Array"), string[] ["Datei Nr.", "Methode Nr.", "Zyklusnr. Mod0", "Zyklusnr. Mod1", "Zyklusnr. Mod2A", "Zyklusnr. Mod2B"], w244, w42, w129, w128, "Probenvolumen1", "Probenvolumen2", "Ventilposition" ("element"), string[] ["CPU Total", "CPU Time critical", "CPU Timed Structures", "CPU High", "CPU Above normal", "CPU Normal", "CPU Background", "CPU Idle", "CPU ISR", "Memory", "SekundenTotalBrutal"]) -> (w246:string[])
      n105 = Build Array (concatenate)(w129, w128) -> (w127:string[])
      n106 = Build Array (concatenate)(w42, w129, w128) -> (w126:string[])
      n107 = Join Numbers(hi=w65, lo=u8 5) -> ((hi.lo)=w62:u16[])
      n108 = Join Numbers(hi=w75, lo=u8 6) -> ((hi.lo)=w73:u16[])
      n109 = Split 1D Array(array=w244, index=2 ("Index")) -> (second subarray=w236:string[])  [unwired: 1 out]
      n110 = Concatenate Strings("HK " ("String"), w78) -> (w82:string)
      n111 = Concatenate Strings("ECD1 " ("String"), w78) -> (w80:string)
      n112 = Concatenate Strings("ECD2 " ("String"), w78) -> (w77:string)
      n113 = property on="dargestellte Größe 1" class="Ring (strikt)"("Strings []"=w126) -> ()  [unwired: 2 in, 2 out]
      n114 = global write "GVZwangs.vi" "ZwangsHorst!"(w147) -> ()
      n115 = global write "GVZwangs.vi" "ZwangsHorst?"(w146) -> ()
      n116 = xnode "Invoke Method"("FPGA-VI-Referenz (Eingang)"=w47, "Daten"=w62) -> ("FPGA-VI-Referenz (Ausgang)"=w68:refnum<k20>)  [unwired: 2 in, 2 out]
      n117 = property on="dargestellte Größe 2" class="Ring (strikt)"("Strings []"=w126) -> ()  [unwired: 2 in, 2 out]
      n118 = property on="dargestellte Größe 3" class="Ring (strikt)"("Strings []"=w127) -> ()  [unwired: 2 in, 2 out]
      n119 = property on="Zeitachse2" class="Ring (strikt)"("Strings []"=w236) -> ()  [unwired: 2 in, 2 out]
      n120 = property on="Zeitachse1" class="Ring (strikt)"("Strings []"=w236) -> ()  [unwired: 2 in, 2 out]
      n121 = xnode "Invoke Method"("FPGA-VI-Referenz (Eingang)"=w68, "Daten"=w73) -> ("FPGA-VI-Referenz (Ausgang)"=w46:refnum<k20>)  [unwired: 2 in, 2 out]
      n122 = Build Path(base path=w85, name or relative path=w82) -> (appended path=w93:path)
      n123 = Build Path(base path=w99, name or relative path=w80) -> (appended path=w95:path)
      n124 = Build Path(base path=w98, name or relative path=w77) -> (appended path=w97:path)
      n125 = global write "GVZwangs.vi" "ZwangsDIO!"(w152) -> ()
      n126 = global write "GVZwangs.vi" "ZwangsDIO?"(w152) -> ()
      n127 = call "MPVSenden_ECD.vi"("Ventilposition"=0, "FPGA-VI-Referenz"=w46) -> ("FPGA-VI-Referenz (Ausgang)"=w44:refnum<k20>)  [unwired: 1 in, 2 out]
      n128 = Create Folder(path (use dialog)=w93) -> (created path=w92:path)  [unwired: 2 in, 2 out]
      n129 = Create Folder(path (use dialog)=w95) -> (created path=w94:path)  [unwired: 2 in, 2 out]
      n130 = Create Folder(path (use dialog)=w97) -> (created path=w96:path)  [unwired: 2 in, 2 out]
      n131 = case shown="True" w116 {
        tunnel: [w271 w276] -> w220
        tunnel: [w271 w275] -> w219
        tunnel: w92 -> [_ w274]
        tunnel: w178 -> [_ w273]
        tunnel: w114 -> [_ w272]
        frame False {
          w271 = refnum<k34> refnum ("tdms1")
        }
        frame True {
          n132 = call "TDMS0.vi"("Startmethode"=w272, "Dateiname"=w273, "Dateiordner"=w274) -> ("tdms1"=w275:refnum<k34>, "tdms0"=w276:refnum<k34>)
          n133 = global write "GVaktuelleTDMS.vi" "aktuelleTDMS-DateiHK"(w276) -> ()
        }
      }
      n134 = case shown="True" w116 {
        tunnel: [w261 w270] -> w218
        tunnel: [w261 w269] -> w217
        tunnel: [w261 w268] -> w216
        tunnel: [w261 w267] -> w215
        tunnel: w94 -> [_ w266]
        tunnel: w177 -> [_ w265]
        tunnel: w96 -> [_ w264]
        tunnel: w176 -> [_ w263]
        tunnel: w114 -> [_ w262]
        frame False {
          w261 = refnum<k34> refnum ("tdms0")
        }
        frame True {
          n135 = call "TDMS0.vi"("Startmethode"=w262, "Dateiname"=w265, "Dateiordner"=w266) -> ("tdms1"=w269:refnum<k34>, "tdms0"=w270:refnum<k34>)
          n136 = call "TDMS0.vi"("Startmethode"=w262, "Dateiname"=w263, "Dateiordner"=w264) -> ("tdms1"=w267:refnum<k34>, "tdms0"=w268:refnum<k34>)
          n137 = global write "GVaktuelleTDMS.vi" "aktuelleTDMS-DateiECD1"(w270) -> ()
          n138 = global write "GVaktuelleTDMS.vi" "aktuelleTDMS-DateiECD2"(w268) -> ()
        }
      }
      n139 = Open/Create/Replace File(file path (use dialog)=path "c:/fromcriocmd.txt" ("Pfad MS-Datei CRIO"), operation (0:open)=T4."replace or create" ("Operation (0:Öffnen)")) -> (refnum out=w212:refnum<file>, error out=w211:errorcluster)  [unwired: 4 in, 1 out]
      n140 = Write to Text File(file (use dialog)=w212, text="time=yyyymmddhhmmss\ncycle=005\ninfo=1234567890123456789012345678901234567890123456789012345678901234567890123456789012345678901234567890\nlength=100\ncmd=cycle" ("Text0 MS-Datei"), error in=w211) -> (refnum out=w209:refnum<file>, error out=w208:errorcluster)  [unwired: 1 in, 1 out]
      n141 = Bundle("created path"=w92, "created path"=w94, "created path"=w96, "Dateiname Housekeeping"=w178, "DateinameECD1"=w177, "DateinameECD2"=w176, "tdms0"=w220, "tdms1"=w219, "tdms0"=w218, "tdms1"=w217, "tdms0"=w216, "tdms1"=w215) -> (w221:T9)  [unwired: 1 in]
      n142 = call "AIKoeffSortieren.vi"("Modul3/AI koeff"=w183, "Modul2/AI koeff"=w184, "Modul1/AI koeff"=w185) -> ("P0"=w224:dbl[], "P1"=w225:dbl[], "P2"=w226:dbl[])
      n143 = Close File(refnum=w209, error in=w208) -> (path=w203:path)  [unwired: 1 out]
      "schnelle Heizungen" <- string[] ["Trap1 [°C]", "Trap2 [°C]", "PreCol1 [°C]", "PreCol2 [°C]", "MainCol1 [°C]", "MainCol2 [°C]"]
    }
    frame #1 {
      w292 = dbl[] [-1.0]
      w361 = 0
      w338 = 0 ("Zyklusnummer1")
      n144 = while {
        stop <- w1051 stop-if-true
        w1045 = 10.0
        n145 = call "Warten2"("Count(mSec)"=u32 1000) -> ()  [unwired: 1 out]
        n146 = global read "gvbooleschRT.vi" "global stop RT"() -> (w1051:bool)
        n147 = global read "GVTrapsMachs.vi" "Traps/Machs"() -> (w1041:dbl[])
        n148 = global read "GVAIs.vi" "AIs"() -> (w1042:dbl[])
        n149 = for {
          N: 9 -> [_]
          shift-right: [w1054] -> w1048
          shift-left: w1042 -> [w1055]
          shift-right: [w1052] -> w1046
          shift-left: w1041 -> [w1053]
          n150 = flat-sequence {
            tunnel: w1055 -> [w1062]
            tunnel: [w1061] -> w1054
            tunnel: w1053 -> [w1060]
            tunnel: [w1059] -> w1052
            frame #0 {
              n151 = call "Warten28"("Count(mSec)"=u32 100) -> ()  [unwired: 1 out]
            }
            frame #1 {
              n152 = global read "GVAIs.vi" "AIs"() -> (w1058:dbl[])
              n153 = Add(x=w1062, y=w1058) -> (x+y=w1061:dbl[])
              n154 = global read "GVTrapsMachs.vi" "Traps/Machs"() -> (w1057:dbl[])
              n155 = Add(x=w1057, y=w1060) -> (x+y=w1059:dbl[])
            }
          }
        }
        n156 = Divide(x=w1048, y=w1045) -> (x/y=w1047:dbl[])
        n157 = Divide(x=w1046, y=w1045) -> (x/y=w1044:dbl[])
        n158 = Build Array (concatenate)(w1047, w1044) -> (w1043:dbl[])
        n159 = global write "GVHK1Hz.vi" "Mod1Mod2Mod3/AITrapsMachs1Hz"(w1043) -> ()
      }
      n160 = while {
        shift-right: ["Methode"] -> _
        shift-left: w387 -> [w1065]
        stop <- w1067 stop-if-true
        n161 = call "Bis zum nächsten Vielfachen warten7"("Count(mSec)"=u32 1000) -> ()  [unwired: 1 out]
        n162 = Not Equal?(x=w1065, y="Methode") -> (x != y?=w1063:bool)
        n163 = global read "gvbooleschRT.vi" "global stop RT"() -> (w1067:bool)
        n164 = global write "GVMethodenwechsel.vi" "Methodenwechsel?"(w1063) -> ()
      }
      n165 = Add Array Elements(numeric array=w312) -> (sum=w311:i32)
      n166 = Array Size(array=w320) -> (size(s)=w341:i32)
      n167 = Unbundle(w337) -> ("created path"=w336:path, "created path"=w334:path, "created path"=w333:path, "Dateiname Housekeeping"=w335:string, "DateinameECD1"=w332:string, "DateinameECD2"=w331:string, "tdms0"=w330:refnum<k34>, "tdms1"=w329:refnum<k34>, "tdms0"=w328:refnum<k34>, "tdms1"=w327:refnum<k34>, "tdms0"=w326:refnum<k34>, "tdms1"=w325:refnum<k34>)
      n168 = Index Array(array=w313, index #1=0 ("Index"), index #2=1 ("Index"), index #3=2 ("Index"), index #4=3 ("Index")) -> (element #1=w350:i32, element #2=w349:i32, element #3=w352:i32, element #4=w351:i32)
      n169 = call <vilib>:"Space Constant.vi"() -> ("String"=w298:string)
      n170 = case shown="True" TRUE ("ECDSpeichern") {
        frame False {
        }
        frame True {
          w558 = dbl[] []
          n171 = global read "GVaktuelleTDMS.vi" "aktuelleTDMS-DateiECD1"() -> (w559:refnum<k34>)
          n172 = while {
            shift-right: [w571] -> _
            shift-left: w558 -> [w575]
            shift-right: [w564] -> _
            shift-left: w558 -> [w568]
            shift-right: [w570] -> _
            shift-left: w559 -> [w573]
            tunnel: w558 -> [w567]
            shift-right: [w561] -> _
            shift-left: errorcluster {"status"=FALSE, "code"=0, "source"=""} ("error IO") -> [w560]
            stop <- w580 stop-if-true
            n173 = call "Bis zum nächsten Vielfachen warten3"("Count(mSec)"=u32 500) -> ()  [unwired: 1 out]
            n174 = global read "GVECDs.vi" "ECD1MW"() -> (w574:dbl[])
            n175 = global read "GVECDs.vi" "ECD2MW"() -> (w565:dbl[])
            n176 = global read "gvbooleschRT.vi" "global stop RT"() -> (w580:bool)
            n177 = Build Array (concatenate)(w575, w574) -> (w572:dbl[])
            n178 = Build Array (concatenate)(w568, w565) -> (w569:dbl[])
            n179 = global read "GVaktuelleTDMS.vi" "aktuelleTDMS-DateiECD1"() -> (w570:refnum<k34>)
            n180 = global read "GVaktuelleTDMS.vi" "aktuelleTDMS-DateiECD2"() -> (w578:refnum<k34>)
            n181 = Equal?(x=w573, y=w570) -> (x = y?=w566:bool)
            n182 = TDMS Write(0:w570, 7:"ECD1", 9:w574, 11:w560) -> (15:w563:errorcluster)  [unwired: 2 in, 3 out]
            n183 = TDMS Write(0:w578, 7:"ECD2", 9:w565, 11:w560) -> (15:w562:errorcluster)  [unwired: 2 in, 3 out]
            n184 = Select(t=w572, s=w566, f=w567) -> (s? t:f=w571:dbl[])
            n185 = Select(t=w569, s=w566, f=w567) -> (s? t:f=w564:dbl[])
            n186 = global write "GVChroms.vi" "ECD1Chrom"(w571) -> ()
            n187 = global write "GVChroms.vi" "ECD2Chrom"(w564) -> ()
            n188 = Merge Errors(w563, w562) -> (w561:errorcluster)
            "TDMSwriteECD" <- w561
          }
        }
      }
      n189 = while {
        shift-right: [w390] -> _
        shift-left: w292 -> [w392]
        shift-right: [w389] -> _
        shift-left: w292 -> [w391]
        stop <- w394 stop-if-true
        n190 = call "Bis zum nächsten Vielfachen warten"("Count(mSec)"=u32 100) -> ()  [unwired: 1 out]
        n191 = case shown="True" "An/Aus" {
          tunnel: w392 -> [w396 w412]
          tunnel: w391 -> [w395 w411]
          tunnel: [w396 w405] -> w390
          tunnel: [w395 w404] -> w389
          frame False {
          }
          frame True {
            w408 = dbl[] [] ("t")
            n192 = global read "GVMWHorst.vi" "MWHorst"() -> (w401:dbl[])
            n193 = global read "GVTrapsMachs.vi" "Traps/Machs"() -> (w402:dbl[])
            n194 = Build Array (concatenate)(w402, w401) -> (w400:dbl[])
            n195 = Index Array(array=w400, index="dargestellte Größe 3") -> (element=w413:dbl)
            n196 = Build Array (concatenate)(w412, w413) -> (w406:dbl[])
            n197 = Select(t=w408, s="TafelWischen!", f=w406) -> (s? t:f=w405:dbl[])
            n198 = global read "GVZeitenZyklen.vi" "Big Ben, Methodenzeit, Zykluszeit0, Zykluszeit1, Zykluszeit2A, Zykluszeit2B"() -> (w399:dbl[])
            n199 = Index Array(array=w399, index=1 ("Index")) -> (element=w397:dbl)
            n200 = Build Array (concatenate)(w411, w397) -> (w407:dbl[])
            n201 = Select(t=w408, s="TafelWischen!", f=w407) -> (s? t:f=w404:dbl[])
            n202 = Bundle(w407, w406) -> (→"schnelleAnzeige":cluster{dbl[], dbl[]})  [unwired: 1 in]
          }
        }
        n203 = global read "gvbooleschRT.vi" "global stop RT"() -> (w394:bool)
      }
      n204 = while {
        tunnel: w316 -> [w618]
        tunnel: w383 -> [w621]
        tunnel: w382 -> [w620]
        tunnel: w381 -> [w619]
        shift-right: [w623] -> _
        shift-left: errorcluster {"status"=FALSE, "code"=0, "source"=""} ("error out") -> [w622]
        stop <- w624 stop-if-true
        n205 = call "AIsFIFORT_ECD.vi"("FPGA-VI-Referenz"=w618, "P2"=w621, "P1"=w620, "P0"=w619, "error in"=w622) -> ("error out"=w623:errorcluster)
        "AIsFIFOread" <- w623
        n206 = global read "gvbooleschRT.vi" "global stop RT"() -> (w624:bool)
      }
      n207 = while {
        tunnel: w316 -> [w625]
        tunnel: w291 -> [w628]
        tunnel: w290 -> [w627]
        tunnel: w289 -> [w626]
        shift-right: [w630] -> _
        shift-left: errorcluster {"status"=FALSE, "code"=0, "source"=""} ("error out") -> [w629]
        stop <- w632 stop-if-true
        n208 = call "Bis zum nächsten Vielfachen warten16"("Count(mSec)"=u32 100) -> ()  [unwired: 1 out]
        n209 = call "TrapsMachMitteln_ECD.vi"("FPGA-VI-Referenz"=w625, "Traps/MachKoeff2"=w628, "Traps/MachKoeff1"=w627, "Traps/MachKoeff0"=w626, "error in"=w629) -> ("error out"=w630:errorcluster)
        "MWTrapsMachs" <- w630
        n210 = global read "gvbooleschRT.vi" "global stop RT"() -> (w632:bool)
      }
      n211 = case shown="True" TRUE ("HKSpeichern") {
        tunnel: w385 -> [_ w611]
        frame False {
        }
        frame True {
          n212 = while {
            tunnel: w611 -> [w615]
            shift-right: [w613] -> _
            shift-left: errorcluster {"status"=FALSE, "code"=0, "source"=""} ("error out") -> [w612]
            stop <- w617 stop-if-true
            n213 = call "Bis zum nächsten Vielfachen warten2"("Count(mSec)"=u32 1000) -> ()  [unwired: 1 out]
            n214 = local read "Methode"() -> (w614:i32)
            n215 = global read "gvbooleschRT.vi" "global stop RT"() -> (w617:bool)
            n216 = call "HKinTDMS-01-16.vi"("Methode"=w614, "error in (no error)"=w612, "Kanäle"=w615) -> ("error out"=w613:errorcluster)
            "TDMSwriteHK" <- w613
          }
        }
      }
      n217 = for {
        N: 1 -> [_]
        tunnel: w316 -> [w633]
        tunnel: [w633] -> w343
        n218 = call "Warten8"("Count(mSec)"=u32 100) -> ()  [unwired: 1 out]
      }
      n219 = Build Array(w298) -> (w297:string[])
      n220 = Initialize Array(-1 ("Element"), 4 ("Dimension")) -> (w314:i32[])
      n221 = global read "GVVentilposition.vi" "Ventilposition"() -> (w322:i32)
      n222 = case shown="True" TRUE {
        tunnel: w338 -> [_ w590]
        tunnel: w336 -> [_ w589]
        tunnel: w335 -> [_ w588]
        tunnel: w330 -> [_ w587]
        tunnel: w329 -> [_ w586]
        frame False {
        }
        frame True {
          w581 = errorcluster {"status"=FALSE, "code"=0, "source"=""} ("error out TDMSopen")
          n223 = while {
            shift-right: [w595] -> w585
            shift-left: w587 -> [w597]
            shift-right: [w606] -> w584
            shift-left: w586 -> [w599]
            shift-right: [w601] -> _
            shift-left: w590 -> [w607]
            tunnel: w588 -> [w603]
            tunnel: w589 -> [w604]
            shift-right: [w594] -> w583
            shift-left: w581 -> [w592]
            shift-right: [w593] -> w582
            shift-left: w581 -> [w591]
            stop <- w609 stop-if-true
            n224 = call "Bis zum nächsten Vielfachen warten5"("Count(mSec)"=u32 500) -> ()  [unwired: 1 out]
            n225 = local read "Methode"() -> (w605:i32)
            n226 = global read "gvbooleschRT.vi" "global stop RT"() -> (w609:bool)
            n227 = global read "GVZeitenZyklen.vi" "ZyklusNummernGesamt"() -> (w596:i32[])
            n228 = Index Array(array=w596, index=1 ("Index")) -> (element=w601:i32)
            n229 = Greater?(x=w601, y=w607) -> (0:w600:bool)
            n230 = Select(t=w599, s=w600, f=w597) -> (s? t:f=w598:refnum<k34>)
            n231 = call "AktuelleTDMS.vi"("AktuelleTDMS"=w597, "error in TDMSopen"=w592, "Dateiordner"=w604, "NächsteTDMS"=w599, "NeuerZyklus?"=w600, "Methodennummer"=w605, "Zyklnumges"=w601, "error in TDMSclose"=w591, "Dateiname"=w603) -> ("AktuelleTDMS"=w595:refnum<k34>, "error out TDMSopen"=w594:errorcluster, "error out TDMSclose"=w593:errorcluster, "NächsteTDMS"=w606:refnum<k34>)  [unwired: 3 in]
            "TDMSopenHK" <- w594
            "TDMScloseHK" <- w593
            n232 = global write "GVaktuelleTDMS.vi" "aktuelleTDMS-DateiHK"(w598) -> ()
          }
          n233 = TDMS Close(8:w583, 11:w585) -> ()  [unwired: 2 out]
          n234 = TDMS Close(8:w582, 11:w584) -> ()  [unwired: 2 out]
        }
      }
      n235 = case shown="True" TRUE {
        tunnel: w338 -> [_ w518]
        tunnel: w334 -> [_ w517]
        tunnel: w333 -> [_ w516]
        tunnel: w332 -> [_ w515]
        tunnel: w331 -> [_ w514]
        tunnel: w328 -> [_ w513]
        tunnel: w327 -> [_ w512]
        tunnel: w326 -> [_ w511]
        tunnel: w325 -> [_ w510]
        frame False {
        }
        frame True {
          w503 = errorcluster {"status"=FALSE, "code"=0, "source"=""} ("error out TDMSopen")
          n236 = while {
            shift-right: [w542] -> w509
            shift-left: w513 -> [w544]
            shift-right: [w552] -> w508
            shift-left: w512 -> [w546]
            shift-right: [w550] -> _
            shift-left: w518 -> [w553]
            tunnel: w517 -> [w549]
            tunnel: w515 -> [w548]
            shift-right: [w541] -> w504
            shift-left: w503 -> [w539]
            shift-right: [w540] -> w505
            shift-left: w503 -> [w538]
            stop <- w555 stop-if-true
            n237 = call "Bis zum nächsten Vielfachen warten4"("Count(mSec)"=u32 500) -> ()  [unwired: 1 out]
            n238 = local read "Methode"() -> (w551:i32)
            n239 = global read "gvbooleschRT.vi" "global stop RT"() -> (w555:bool)
            n240 = global read "GVZeitenZyklen.vi" "ZyklusNummernGesamt"() -> (w543:i32[])
            n241 = Index Array(array=w543, index=2 ("Index")) -> (element=w550:i32)
            n242 = Greater?(x=w550, y=w553) -> (0:w547:bool)
            n243 = Select(t=w546, s=w547, f=w544) -> (s? t:f=w545:refnum<k34>)
            n244 = call "AktuelleTDMS.vi"("AktuelleTDMS"=w544, "error in TDMSopen"=w539, "Dateiordner"=w549, "NächsteTDMS"=w546, "NeuerZyklus?"=w547, "Methodennummer"=w551, "Zyklnumges"=w550, "error in TDMSclose"=w538, "Dateiname"=w548) -> ("AktuelleTDMS"=w542:refnum<k34>, "error out TDMSopen"=w541:errorcluster, "error out TDMSclose"=w540:errorcluster, "NächsteTDMS"=w552:refnum<k34>)  [unwired: 3 in]
            "TDMSopenECD1" <- w541
            "TDMScloseECD1" <- w540
            n245 = global write "GVaktuelleTDMS.vi" "aktuelleTDMS-DateiECD1"(w545) -> ()
          }
          n246 = while {
            shift-right: [w532] -> w507
            shift-left: w511 -> [w524]
            shift-right: [w533] -> w506
            shift-left: w510 -> [w526]
            shift-right: [w530] -> _
            shift-left: w518 -> [w534]
            tunnel: w516 -> [w529]
            tunnel: w514 -> [w528]
            shift-right: [w522] -> _
            shift-left: w503 -> [w520]
            shift-right: [w521] -> _
            shift-left: w503 -> [w519]
            stop <- w536 stop-if-true
            n247 = call "Bis zum nächsten Vielfachen warten6"("Count(mSec)"=u32 500) -> ()  [unwired: 1 out]
            n248 = local read "Methode"() -> (w531:i32)
            n249 = global read "gvbooleschRT.vi" "global stop RT"() -> (w536:bool)
            n250 = global read "GVZeitenZyklen.vi" "ZyklusNummernGesamt"() -> (w523:i32[])
            n251 = Index Array(array=w523, index=3 ("Index")) -> (element=w530:i32)
            n252 = Greater?(x=w530, y=w534) -> (0:w527:bool)
            n253 = Select(t=w526, s=w527, f=w524) -> (s? t:f=w525:refnum<k34>)
            n254 = call "AktuelleTDMS.vi"("AktuelleTDMS"=w524, "error in TDMSopen"=w520, "Dateiordner"=w529, "NächsteTDMS"=w526, "NeuerZyklus?"=w527, "Methodennummer"=w531, "Zyklnumges"=w530, "error in TDMSclose"=w519, "Dateiname"=w528) -> ("AktuelleTDMS"=w532:refnum<k34>, "error out TDMSopen"=w522:errorcluster, "error out TDMSclose"=w521:errorcluster, "NächsteTDMS"=w533:refnum<k34>)  [unwired: 3 in]
            "TDMSopenECD2" <- w522
            "TDMScloseECD2" <- w521
            n255 = global write "GVaktuelleTDMS.vi" "aktuelleTDMS-DateiECD2"(w525) -> ()
          }
          n256 = TDMS Close(8:w504, 11:w509) -> ()  [unwired: 2 out]
          n257 = TDMS Close(8:w505, 11:w508) -> ()  [unwired: 2 out]
          n258 = TDMS Close(11:w507) -> ()  [unwired: 1 in, 2 out]
          n259 = TDMS Close(11:w506) -> ()  [unwired: 1 in, 2 out]
        }
      }
      n260 = Add(x=w352, y=w351) -> (x+y=w348:i32)
      n261 = Bundle(w297, w297, w297) -> (w359:cluster{string[], string[], string[]})  [unwired: 1 in]
      n262 = Index Array(array=w307, index=w305) -> (element=w306:T7)
      n263 = Initialize Array(cluster{"output high":dbl, "output low":dbl} {"output high"=99999.0, "output low"=0.0} ("output range"), w341) -> (w321:cluster{"output high":dbl, "output low":dbl}[])
      n264 = Concatenate Strings("?SE0,GDATA" ("Schreibpuffer"), "\r") -> (w293:string)
      n265 = Build Array(w350, w349, w348) -> (w282:i32[])
      n266 = while {
        tunnel: w386 -> [w746]
        shift-right: [w745] -> _
        shift-left: w307 -> [w727]
        tunnel: w321 -> [w744]
        tunnel: w320 -> [w743]
        tunnel: w316 -> [w742]
        tunnel: w319 -> [w741]
        tunnel: w318 -> [w740]
        shift-right: [w734] -> _
        shift-left: 0 -> [w739]
        tunnel: w316 -> [w738]
        tunnel: w315 -> [w737]
        shift-right: [w733] -> _
        shift-left: w314 -> [w736]
        tunnel: w313 -> [w728]
        tunnel: w312 -> [w729]
        tunnel: w311 -> [w730]
        tunnel: w310 -> [w731]
        tunnel: w309 -> [w732]
        tunnel: w308 -> [w735]
        shift-right: [w650] -> _
        shift-left: w306 -> [w649]
        tunnel: w291 -> [w635]
        tunnel: w290 -> [w636]
        tunnel: w289 -> [w637]
        tunnel: w284 -> [w638]
        i -> [w653]
        stop <- w747 stop-if-true
        w643 = 0  # ZeileMainMach2
        w644 = 0  # ZeileMainMach1
        w695 = FALSE
        w694 = 0.0
        w696 = 0  # ZeilennummerMPV
        w700 = cluster{dbl[], dbl[]} {[], []}
        w709 = dbl[] []
        w713 = 0  # ZeilePreMach2
        w714 = 0  # ZeilePreMach1
        w715 = 0  # ZeileFPGAFixp
        w716 = 0  # ZeileFPGAPID
        w717 = 0  # ZeileFPGABoolesch
        w718 = i32[] [0, 0, 0, 0]  # ZeilennummernHorst
        w719 = i32[] [0, 0, 0, 0]  # ZeilennummernDIOs
        n267 = Unbundle(w649) -> ("Zykluslängen [s]"=w693:dbl[], "ZeitpktDIOsMod0"=w692:dbl[], "ZeitpktDIOsMod1"=w691:dbl[], "ZeitpktDIOsMod2A"=w690:dbl[], "ZeitpktDIOsMod2B"=w689:dbl[], "DIOsSPMod0"=w688:bool[][], "DIOsSPMod1"=w687:bool[][], "DIOsSPMod2A"=w686:bool[][], "DIOsSPMod2B"=w685:bool[][], "Mod0HorstZeitpkt"=w684:dbl[], "Mod1HorstZeitpkt"=w683:dbl[], "Mod2AHorstZeitpkt"=w682:dbl[], "Mod2BHorstZeitpkt"=w681:dbl[], "HorstSPMod0"=w680:dbl[][], "HorstSPMod1"=w679:dbl[][], "HorstSPMod2A"=w678:dbl[][], "HorstSPMod2B"=w677:dbl[][], "LHSetpoints"=w676:dbl[], "LHHeizen?"=w675:bool[], "ZPktFPGABoolesch"=w674:dbl[], "FPGABoolesch"=w673:bool[][], "ZeitpktFPGAPID"=w672:dbl[], "FPGAPID"=w671:T10, "ZeitpktFPGAFixp"=w670:dbl[], w669:dbl[][], "t_PreMach1"=w668:dbl[], "T_PreMach1"=w667:dbl[], "t_PreMach2"=w666:dbl[], "T_PreMach2"=w665:dbl[], "PIDs für \"träge\" Heizungen"=w664:T11, "Zwangsbedingungen"=w663:dbl[][], "Dateien fürs MS schicken?"=w662:bool, "ZeitpunkteMPV"=w661:dbl[], "SPMPV"=w660:i32[], "ZeitpktMS-1"=w659:dbl, "ZeitpktMS-2"=w658:dbl, "Int.Start1"=w657:dbl, "Int.Stop1"=w656:dbl, "Int.Start2"=w655:dbl, "Int.Stop2"=w654:dbl, "t_MainMach1"=w648:dbl[], "T_MainMach1"=w647:dbl[], "t_MainMach2"=w646:dbl[], "T_MainMach2"=w645:dbl[])  [unwired: 1 out]
        n268 = Add(x=w736, y=1) -> (x+y=w704:i32[])
        n269 = local read "Methode"() -> (w652:i32)
        n270 = while {
          tunnel: w729 -> [w816]
          tunnel: w732 -> [w809]
          tunnel: w731 -> [w810]
          tunnel: w728 -> [w815]
          tunnel: w730 -> [w811]
          tunnel: w663 -> [w812]
          stop <- w818 stop-if-true
          n271 = call "Bis zum nächsten Vielfachen warten10"("Count(mSec)"=u32 1000) -> ()  [unwired: 1 out]
          n272 = local read "Methode"() -> (w814:i32)
          n273 = global read "GVMethodenwechsel.vi" "Methodenwechsel?"() -> (w820:bool)
          n274 = global read "gvbooleschRT.vi" "global stop RT"() -> (w821:bool)
          n275 = case shown="True" "global stop RT" {
            frame False {
            }
            frame True {
              n276 = global write "gvbooleschRT.vi" "global stop RT"(TRUE ("global stop RT")) -> ()
            }
          }
          n277 = call "ZwangsbedingungenGV-15-07-17.vi"("AnzahlHorst"=w809, "AnzahlHorst/Modul"=w815, "AnzahlLH"=w810, "AnzahlDIOs/Modul"=w816, "AnzahlDIOs"=w811, "Zwangsbedingungen"=w812, "Methodennummer"=w814) -> ("Methodennummer"=w813:i32)  [unwired: 4 in]
          n278 = local write "Methode"(w813) -> ()
          n279 = local read "veränderte Methode benutzen"() -> (w819:bool)
          n280 = Compound Arithmetic op=OR(w821, w820, w819) -> (w818:bool)
        }
        n281 = Build Cluster Array(w688, w687, w686, w685) -> (w723:cluster{"DIOsSPMod2B":bool[][]}[])
        n282 = Build Cluster Array(w680, w679, w678, w677) -> (w721:cluster{"HorstSPMod2B":dbl[][]}[])
        n283 = Build Cluster Array(w692, w691, w690, w689) -> (w724:cluster{"ZeitpktDIOsMod2B":dbl[]}[])
        n284 = Build Cluster Array(w684, w683, w682, w681) -> (w722:cluster{"Mod2BHorstZeitpkt":dbl[]}[])
        n285 = Equal?(x=w653, y=0) -> (x = y?=w725:bool)
        n286 = global read "GVZeitenZyklen.vi" "ZyklusNummern"() -> (w703:i32[])
        n287 = global read "GVZwangs.vi" "ZwangsHorst?"() -> (w708:cluster{bool[]}[])
        n288 = global read "gvbooleschRT.vi" "global stop RT"() -> (w747:bool)
        n289 = global read "GVZwangsMPV.vi" "ZwangsMPV?"() -> (w641:bool)
        n290 = global read "GVZwangs.vi" "ZwangsDIO?"() -> (w707:cluster{bool[]}[])
        n291 = global read "GVaktuelleTDMS.vi" "aktuelleTDMS-DateiECD1"() -> (w702:refnum<k34>)
        n292 = while {
          tunnel: w743 -> [w799]
          tunnel: w744 -> [w802]
          tunnel: w742 -> [w803]
          tunnel: w676 -> [w800]
          tunnel: w664 -> [w801]
          shift-right: [w797] -> _
          shift-left: errorcluster {"status"=FALSE, "code"=0, "source"=""} ("error out") -> [w798]
          stop <- w804 stop-if-true
          n293 = call "LH_ECD.vi"("FPGA-VI-Referenz"=w803, "OutputRange"=w802, "LHSetpoints"=w800, "AIsLH"=w799, "error in"=w798, "LH-Gruppe"="LH-Gruppe", "PIDs für \"träge\" Heizungen"=w801) -> ("error out"=w797:errorcluster)
          "LH" <- w797
          n294 = call "Bis zum nächsten Vielfachen warten12"("Count(mSec)"=u32 100) -> ()  [unwired: 1 out]
          n295 = global read "GVMethodenwechsel.vi" "Methodenwechsel?"() -> (w806:bool)
          n296 = global read "gvbooleschRT.vi" "global stop RT"() -> (w807:bool)
          n297 = local read "veränderte Methode benutzen"() -> (w805:bool)
          n298 = Compound Arithmetic op=OR(w807, w806, w805) -> (w804:bool)
        }
        n299 = while {
          shift-right: [w760] -> _
          shift-left: w695 -> [w764]
          shift-right: [w759] -> _
          shift-left: w694 -> [w763]
          shift-right: [w758] -> _
          shift-left: w695 -> [w762]
          shift-right: [w757] -> _
          shift-left: w694 -> [w761]
          tunnel: w735 -> [w756]
          tunnel: w657 -> [w751]
          tunnel: w656 -> [w750]
          tunnel: w655 -> [w749]
          tunnel: w654 -> [w748]
          stop <- w753 stop-if-true
          n300 = call "Integrieren.vi"("Integrieren1"=w764, "Integral1"=w763, "Integrieren2"=w762, "Integral2"=w761, "Int.Start1"=w751, "Int.Stop1"=w750, "Int.Start2"=w749, "HorstProbenflußNr."=w756, "Int.Stop2"=w748) -> ("Integrieren1"=w760:bool, "Integral1"=w759:dbl, "Integrieren2"=w758:bool, "Integral2"=w757:dbl)  [unwired: 7 in]
          n301 = call "Bis zum nächsten Vielfachen warten9"("Count(mSec)"=u32 100) -> ()  [unwired: 1 out]
          n302 = global read "GVMethodenwechsel.vi" "Methodenwechsel?"() -> (w754:bool)
          n303 = global read "gvbooleschRT.vi" "global stop RT"() -> (w755:bool)
          n304 = local read "veränderte Methode benutzen"() -> (w752:bool)
          n305 = Compound Arithmetic op=OR(w755, w754, w752) -> (w753:bool)
        }
        n306 = while "Zeit" {
          tunnel: w725 -> [w1002]
          tunnel: w693 -> [w1000]
          tunnel: w704 -> [w995]
          tunnel: [w994] -> w733
          shift-right: [w991] -> _
          shift-left: 0.0 -> [w992]
          i -> [w1004]
          stop <- w997 stop-if-true
          n307 = Equal?(x=w1004, y=0) -> (x = y?=w993:bool)
          n308 = call "Bis zum nächsten Vielfachen warten15"("Count(mSec)"=u32 50) -> ()  [unwired: 1 out]
          n309 = call "BigBen_ECD.vi"("MethodenStartzeit"=w992, "Methodenstart?"=w993, "Programmstart?"=w1002, "Zykluslängen [s]"=w1000, "MethodenStartZyklusNummern"=w995) -> ("MethodenStartzeit"=w991:dbl, "ZyklusNummernGesamt"=w994:i32[])  [unwired: 2 in]
          n310 = global read "GVMethodenwechsel.vi" "Methodenwechsel?"() -> (w996:bool)
          n311 = global read "gvbooleschRT.vi" "global stop RT"() -> (w1001:bool)
          n312 = Or(x=w996, y=w1001) -> (x .or. y?=w998:bool)
          n313 = local read "veränderte Methode benutzen"() -> (w999:bool)
          n314 = Or(x=w999, y=w998) -> (x .or. y?=w997:bool)
        }
        n315 = Bundle(w724, w723, w722, w721, "LHHeizen?"=w675, "ZPktFPGABoolesch"=w674, "FPGABoolesch"=w673, "ZeitpktFPGAPID"=w672, "FPGAPID"=w671, "ZeitpktFPGAFixp"=w670, w669, "t_PreMach1"=w668, "T_PreMach1"=w667, "t_PreMach2"=w666, "T_PreMach2"=w665, "ZeitpunkteMPV"=w661, "SPMPV"=w660, "t_MainMach1"=w648, "T_MainMach1"=w647, "t_MainMach2"=w646, "T_MainMach2"=w645) -> (w720:T12)  [unwired: 1 in]
        n316 = Index Array(array=w727, index=w652) -> (element=w651:T7)
        n317 = global read "GVZwangs.vi" "ZwangsFPGABoolesch?"() -> (w706:bool[])
        n318 = while {
          tunnel: w746 -> [w1017]
          shift-right: [w1008] -> _
          shift-left: w651 -> [w1016]
          tunnel: w652 -> [w1014]
          shift-right: [w1006] -> w745
          shift-left: w727 -> [w1015]
          tunnel: [w1007] -> w650
          stop <- w1010 stop-if-true
          n319 = call "Bis zum nächsten Vielfachen warten8"("Count(mSec)"=u32 500) -> ()  [unwired: 1 out]
          n320 = global read "GVMethodenwechsel.vi" "Methodenwechsel?"() -> (w1012:bool)
          n321 = global read "gvbooleschRT.vi" "global stop RT"() -> (w1011:bool)
          n322 = case shown="True" "Methode verändern" {
            tunnel: w1017 -> [_ w1039]
            tunnel: w1016 -> [w1036 w1038]
            tunnel: [w1036 w1037] -> w1008
            frame False {
            }
            frame True {
              n323 = call "methodeändern-15-07-17.vi"("->Methode"=w1038, "Namen"=w1039) -> ("Methode->"=w1037:T13)  [unwired: 1 in]
              n324 = property on="Methode verändern" class="Bool. (strikt)"("Value"=FALSE ("Methode verändern")) -> ()  [unwired: 2 in, 2 out]
            }
          }
          n325 = Compound Arithmetic op=OR(w1012, w1011, "veränderte Methode benutzen") -> (w1010:bool)
          n326 = case shown="True" "Methode speichern" {
            tunnel: w1008 -> [_ w1033]
            tunnel: w1015 -> [w1026 w1035]
            tunnel: w1014 -> [_ w1034]
            tunnel: [w1026 w1028] -> w1006
            frame False {
            }
            frame True {
              n327 = Replace Array Subset(array=w1035, new element=w1033, index=w1034) -> (w1028:T3)
              n328 = property on="Methode speichern" class="Bool. (strikt)"("Value"=FALSE ("Methode speichern")) -> ()  [unwired: 2 in, 2 out]
              n329 = Open/Create/Replace File(file path (use dialog)=path "c:/methoden.pery" ("Dateipfad (Dialog verwenden)"), operation (0:open)=T4."replace" ("Operation (0:Öffnen)")) -> (refnum out=w1030:refnum<file>)  [unwired: 4 in, 2 out]
              n330 = Write to Binary File(file (use dialog)=w1030, data=w1028) -> (refnum out=w1027:refnum<file>)  [unwired: 4 in, 2 out]
              n331 = Close File(refnum=w1027) -> ()  [unwired: 1 in, 2 out]
            }
          }
          n332 = case shown="False" "veränderte Methode benutzen" {
            tunnel: w1008 -> [_ w1023]
            tunnel: [w1020 w1023] -> w1007
            tunnel: w1006 -> [w1022 _]
            frame False {
              n333 = local read "Methode"() -> (w1021:i32)
              n334 = Index Array(array=w1022, index=w1021) -> (element=w1020:T7)
            }
            frame True {
              n335 = flat-sequence {
                frame #0 {
                  n336 = call "Warten"("Count(mSec)"=u32 1100) -> ()  [unwired: 1 out]
                }
                frame #1 {
                  n337 = property on="veränderte Methode benutzen" class="Bool. (strikt)"("Value"=FALSE ("Methode verändern")) -> ()  [unwired: 2 in, 2 out]
                }
              }
            }
          }
        }
        n338 = Bundle(w709, w709, w709, w709) -> (w710:cluster{dbl[], dbl[], dbl[], dbl[]})  [unwired: 1 in]
        n339 = Bundle("ZyklusNummern"=w703, "ZeilennummernDIOs"=w719, "ZwangsDIO?"=w707, "ZeilennummernHorst"=w718, "ZwangsHorst?"=w708, "ZeileFPGABoolesch"=w717, "ZwangsFPGABoolesch?"=w706, "ZeileFPGAPID"=w716, "ZeileFPGAFixp"=w715, "ZeilePreMach1"=w714, "ZeilePreMach2"=w713, "ZeilennummerMPV"=w696, "ZeileMainMach1"=w644, "ZeileMainMach2"=w643, "ZwangsMPV?"=w641) -> (w712:T14)  [unwired: 1 in]
        n340 = while {
          shift-right: [w934] -> _
          shift-left: w710 -> [w941]
          shift-right: [w933] -> _
          shift-left: w710 -> [w940]
          shift-right: [w931] -> _
          shift-left: T5 {"Zyklus1"=0, "Zeitachse1"=0, "dargestellte Größe 1"=0, "Zyklus2"=0, "Zeitachse2"=0, "dargestellte Größe 2"=0} ("AnzeigeEinstellungen") -> [w939]
          tunnel: w693 -> [w909]
          shift-right: [w905] -> _
          shift-left: w702 -> [w904]
          shift-right: [w900] -> _
          shift-left: w700 -> [w902]
          shift-right: [w889] -> _
          shift-left: w700 -> [w901]
          shift-right: ["Detektor"] -> _
          shift-left: 0 ("Detektor") -> [w898]
          tunnel: w638 -> [w887]
          stop <- w945 stop-if-true
          w910 = 0.0 ("X-Achse.Bereich:Minimum")
          n341 = Unbundle(w887) -> ("Modul1/AI sicherer Bereich"=w880:dbl[][], "Modul2/AI sicherer Bereich"=w865:dbl[][], "Modul3/AI sicherer Bereich"=w856:dbl[][], "Traps/Machs sicherer Bereich"=w847:dbl[][], w839:dbl[][], "Metavariablen grüner Bereich"=w830:dbl[][])
          n342 = call "Bis zum nächsten Vielfachen warten14"("Count(mSec)"=u32 1000) -> ()  [unwired: 1 out]
          n343 = global read "GVMWHorst.vi" "MWHorst"() -> (w838:dbl[])
          "MWHorst" <- w838
          n344 = case shown="0, Standard" "Detektor" {
            tunnel: [w955 w967] -> w900
            tunnel: w909 -> [w954 w969]
            tunnel: "Detektor" -> [w949 w963]
            tunnel: [w953 w968] -> w907
            tunnel: [w952 w966] -> w905
            frame 0, Default {
              n345 = Increment(x=w949) -> (x+1=w950:i32)
              n346 = Increment(x=w950) -> (x+1=w948:i32)
              n347 = global read "GVChroms.vi" "ECD1Chrom"() -> (w951:dbl[])
              n348 = global read "GVaktuelleTDMS.vi" "aktuelleTDMS-DateiECD1"() -> (w952:refnum<k34>)
              n349 = Index Array(array=w954, index=w948) -> (element=w953:dbl)
              n350 = Array Size(array=w951) -> (size(s)=w957:i32)
              n351 = for {
                N: w957 -> [_]
                tunnel: [w958] -> w956 mode=indexing
                i -> [w961]
                n352 = To Double Precision Float(number=w961) -> (double precision float=w960:dbl)
                n353 = Divide(x=w960, y=10.0) -> (x/y=w958:dbl)
              }
              n354 = Bundle(w956, "ECD1Chrom"=w951) -> (w955:cluster{dbl[], "ECD1Chrom":dbl[]})  [unwired: 1 in]
            }
            frame 1 {
              n355 = Increment(x=w963) -> (x+1=w964:i32)
              n356 = Increment(x=w964) -> (x+1=w962:i32)
              n357 = global read "GVChroms.vi" "ECD2Chrom"() -> (w965:dbl[])
              n358 = global read "GVaktuelleTDMS.vi" "aktuelleTDMS-DateiECD2"() -> (w966:refnum<k34>)
              n359 = Index Array(array=w969, index=w962) -> (element=w968:dbl)
              n360 = Array Size(array=w965) -> (size(s)=w971:i32)
              n361 = for {
                N: w971 -> [_]
                tunnel: [w972] -> w970 mode=indexing
                i -> [w975]
                n362 = To Double Precision Float(number=w975) -> (double precision float=w974:dbl)
                n363 = Divide(x=w974, y=10.0) -> (x/y=w972:dbl)
              }
              n364 = Bundle(w970, "ECD2Chrom"=w965) -> (w967:cluster{dbl[], "ECD2Chrom":dbl[]})  [unwired: 1 in]
            }
          }
          n365 = Subtract(x="DetYMax", y="DetYMin") -> (x-y=w915:dbl)
          n366 = Subtract(x="HK1YMax", y="HK1YMin") -> (x-y=w925:dbl)
          n367 = Subtract(x="HK2YMax", y="HK2YMin") -> (x-y=w920:dbl)
          n368 = Equal?(x="Detektor", y=w898) -> (x = y?=w897:bool)
          n369 = Index Array(array=w880, index (col) #1=0 ("disabled index (col)"), index (col) #2=1 ("index (col)")) -> (element #1=w877:dbl[], element #2=w875:dbl[])  [unwired: 2 in]
          n370 = Index Array(array=w865, index (col) #1=0 ("disabled index (col)"), index (col) #2=1 ("index (col)")) -> (element #1=w869:dbl[], element #2=w868:dbl[])  [unwired: 2 in]
          n371 = Index Array(array=w847, index (col) #1=0 ("disabled index (col)"), index (col) #2=1 ("index (col)")) -> (element #1=w851:dbl[], element #2=w850:dbl[])  [unwired: 2 in]
          n372 = Index Array(array=w839, index (col) #1=0 ("disabled index (col)"), index (col) #2=1 ("index (col)")) -> (element #1=w843:dbl[], element #2=w842:dbl[])  [unwired: 2 in]
          n373 = Index Array(array=w856, index (col) #1=0 ("disabled index (col)"), index (col) #2=1 ("index (col)")) -> (element #1=w860:dbl[], element #2=w859:dbl[])  [unwired: 2 in]
          n374 = Index Array(array=w830, index (col) #1=0 ("disabled index (col)"), index (col) #2=1 ("index (col)")) -> (element #1=w834:dbl[], element #2=w833:dbl[])  [unwired: 2 in]
          n375 = global read "GVMethodenwechsel.vi" "Methodenwechsel?"() -> (w943:bool)
          n376 = global read "GVZeitenZyklen.vi" "ZyklusNummern"() -> (w912:i32[])
          "ZyklusNummern" <- w912
          n377 = global read "gvbooleschRT.vi" "global stop RT"() -> (w944:bool)
          n378 = global read "GVMetavariablen.vi" "Metavariablen"() -> (w829:dbl[])
          "Metavariablen" <- w829
          n379 = global read "GVVentilposition.vi" "Ventilposition"() -> (→"Ventilposition":i32)
          n380 = global read "GVZeitenZyklen.vi" "ZyklusNummernGesamt"() -> (→"ZyklusNummernGesamt":i32[])
          n381 = Divide(x=w915, y=20.0) -> (x/y=w913:dbl)
          n382 = Divide(x=w925, y=10.0) -> (x/y=w923:dbl)
          n383 = Divide(x=w920, y=10.0) -> (x/y=w918:dbl)
          n384 = local read "veränderte Methode benutzen"() -> (w942:bool)
          n385 = Or(x=w943, y=w944) -> (x .or. y?=w946:bool)
          n386 = Greater Or Equal?(x=w838, y=w843) -> (x >= y?=w841:bool[])
          n387 = Less Or Equal?(x=w838, y=w842) -> (x <= y?=w840:bool[])
          n388 = Greater Or Equal?(x=w829, y=w834) -> (x >= y?=w832:bool[])
          n389 = Less Or Equal?(x=w829, y=w833) -> (x <= y?=w831:bool[])
          n390 = global read "GVHK1Hz.vi" "Mod1Mod2Mod3/AITrapsMachs1Hz"() -> (w825:dbl[])
          n391 = And(x=w841, y=w840) -> (x .and. y?=→"HorstOK?":bool[])
          n392 = And(x=w832, y=w831) -> (x .and. y?=→"MVOK?":bool[])
          n393 = Or(x=w946, y=w942) -> (x .or. y?=w945:bool)
          n394 = global read "GVZeitenZyklen.vi" "Big Ben, Methodenzeit, Zykluszeit0, Zykluszeit1, Zykluszeit2A, Zykluszeit2B"() -> (w892:dbl[])
          n395 = Array Subset(array=w825, index=0 ("Index"), length=32 ("Länge")) -> (w876:dbl[])
          "AIs1" <- w876
          n396 = Array Subset(array=w825, index=32 ("Index"), length=32 ("Länge")) -> (w864:dbl[])
          "AIs2" <- w864
          n397 = Array Subset(array=w825, index=96 ("Index"), length=6 ("Länge")) -> (w824:dbl[])
          "schnelle Heizungen" <- w824
          n398 = Array Subset(array=w825, index=64 ("Index"), length=32 ("Länge")) -> (w855:dbl[])
          "AIs3" <- w855
          n399 = Greater Or Equal?(x=w824, y=w851) -> (x >= y?=w849:bool[])
          n400 = Less Or Equal?(x=w824, y=w850) -> (x <= y?=w848:bool[])
          n401 = Greater Or Equal?(x=w876, y=w877) -> (x >= y?=w874:bool[])
          n402 = Less Or Equal?(x=w876, y=w875) -> (x <= y?=w873:bool[])
          n403 = Greater Or Equal?(x=w864, y=w869) -> (x >= y?=w867:bool[])
          n404 = Less Or Equal?(x=w864, y=w868) -> (x <= y?=w866:bool[])
          n405 = And(x=w849, y=w848) -> (x .and. y?=→"SHOK?":bool[])
          n406 = Greater Or Equal?(x=w855, y=w860) -> (x >= y?=w858:bool[])
          n407 = Less Or Equal?(x=w855, y=w859) -> (x <= y?=w857:bool[])
          n408 = And(x=w874, y=w873) -> (x .and. y?=→"AIs1OK?":bool[])
          n409 = And(x=w867, y=w866) -> (x .and. y?=→"AIs2OK?":bool[])
          n410 = And(x=w858, y=w857) -> (x .and. y?=→"AIs3OK?":bool[])
          n411 = To Long Integer(number=w892) -> (32bit integer=→"Big Ben, Methodenzeit, Zykluszeit0, Zykluszeit1, Zykluszeit2A, Zykluszeit2B":i32[])
          n412 = Equal?(x=w905, y=w904) -> (x = y?=w903:bool)
          n413 = call "AnzeigeGV.vi"("veränderte Methode benutzen"=w942, "Zykluslängen [s]"=w909, "Cluster1"=w941, "Big Ben, Methodenzeit, Zykluszeit0, Zykluszeit1, Zykluszeit2A, Zykluszeit2B"=w892, "Zyklusnummern 0, 1, 2A, 2B"=w912, "Cluster2"=w940, "AnzeigeEinstellungen"=w939, "dargestellte Größe 1"="dargestellte Größe 1", "Zeitachse1"="Zeitachse1", "dargestellte Größe 2"="dargestellte Größe 2", "Zeitachse2"="Zeitachse2") -> ("Anzeige2"=→"Housekeeping2":cluster{dbl[], dbl[]}, "Cluster1"=w934:cluster{dbl[], dbl[], dbl[], dbl[]}, "x1Inkr"=w929:dbl, "Cluster2"=w933:cluster{dbl[], dbl[], dbl[], dbl[]}, "Anzeige1"=→"Housekeeping1":cluster{dbl[], dbl[]}, "AnzeigeEinstellungen"=w931:T5, "x2Max"=w893:dbl, "x2Inkr"=w928:dbl, "x1Max"=w894:dbl)  [unwired: 8 in]
          n414 = Divide(x=w907, y=20.0) -> (x/y=w908:dbl)
          n415 = property on="Detektor 2" class="XYGraph (strikt)"("XScale.Minimum"=w910, "XScale.Maximum"=w907, "XScale.Increment"=w908, "YScale.Minimum"="DetYMin", "YScale.Maximum"="DetYMax", "YScale.Increment"=w913) -> ()  [unwired: 2 in, 2 out]
          n416 = property on="Housekeeping1" class="XYGraph (strikt)"("XScale.Minimum"=w910, "XScale.Maximum"=w894, "XScale.Increment"=w929, "YScale.Minimum"="HK1YMin", "YScale.Maximum"="HK1YMax", "YScale.Increment"=w923) -> ()  [unwired: 2 in, 2 out]
          n417 = property on="Housekeeping2" class="XYGraph (strikt)"("XScale.Minimum"=w910, "XScale.Maximum"=w893, "XScale.Increment"=w928, "YScale.Minimum"="HK2YMin", "YScale.Maximum"="HK2YMax", "YScale.Increment"=w918) -> ()  [unwired: 2 in, 2 out]
          n418 = Select(t=w901, s=w903, f=w902) -> (s? t:f=w896:cluster{dbl[], dbl[]})
          n419 = Select(t=w896, s=w897, f=cluster{dbl[], dbl[]} {[], []} ("s? t:f")) -> (s? t:f=w889:cluster{dbl[], dbl[]})
          n420 = Build Array(w900, w889) -> (→"Detektor 2":cluster{dbl[], "ECD2Chrom":dbl[]}[])
        }
        n421 = while "ZyklusSteuerung" {
          tunnel: w737 -> [w980]
          tunnel: w738 -> [w976]
          shift-right: [w978] -> _
          shift-left: w712 -> [w984]
          tunnel: w720 -> [w985]
          tunnel: w637 -> [w981]
          tunnel: w636 -> [w982]
          tunnel: w635 -> [w983]
          shift-right: [w977] -> _
          shift-left: errorcluster {"status"=FALSE, "code"=0, "source"=""} ("error out") -> [w979]
          stop <- w986 stop-if-true
          n422 = call "Bis zum nächsten Vielfachen warten11"("Count(mSec)"=u32 100) -> ()  [unwired: 1 out]
          n423 = global read "GVMethodenwechsel.vi" "Methodenwechsel?"() -> (w989:bool)
          n424 = global read "gvbooleschRT.vi" "global stop RT"() -> (w988:bool)
          n425 = local read "veränderte Methode benutzen"() -> (w987:bool)
          n426 = Compound Arithmetic op=OR(w989, w988, w987) -> (w986:bool)
          n427 = call "ZyklussteuerungGV_ECD.vi"("Traps/MachKoeff0"=w981, "DIOsNummern"=w980, "error in"=w979, "Traps/MachKoeff1"=w982, "FPGA-VI-Referenz"=w976, "Traps/MachKoeff2"=w983, "Schieberegister"=w984, "Zeitpunkte/Setpoints"=w985) -> ("Schieberegister"=w978:T15, "error out"=w977:errorcluster)  [unwired: 6 in]
          "Zyklus" <- w977
        }
        n428 = global read "GVZeitenZyklen.vi" "Big Ben, Methodenzeit, Zykluszeit0, Zykluszeit1, Zykluszeit2A, Zykluszeit2B"() -> (w699:dbl[])
        n429 = Index Array(array=w699, index=3 ("Index")) -> (element=w697:dbl)
        n430 = while {
          tunnel: w741 -> [w768]
          tunnel: w740 -> [w767]
          tunnel: w662 -> [w782]
          shift-right: [w783] -> w734
          shift-left: w739 -> [w784]
          tunnel: w659 -> [w778]
          tunnel: w658 -> [w772]
          shift-right: [w769] -> _
          shift-left: w697 -> [w773]
          stop <- w785 stop-if-true
          n431 = Less?(x=w773, y=w778) -> (x < y?=w776:bool)
          n432 = Less?(x=w773, y=w772) -> (x < y?=w774:bool)
          n433 = call "Bis zum nächsten Vielfachen warten13"("Count(mSec)"=u32 100 ("Zu wartende ms")) -> ()  [unwired: 1 out]
          n434 = global read "GVMethodenwechsel.vi" "Methodenwechsel?"() -> (w787:bool)
          n435 = global read "gvbooleschRT.vi" "global stop RT"() -> (w788:bool)
          n436 = local read "veränderte Methode benutzen"() -> (w786:bool)
          n437 = Compound Arithmetic op=OR(w788, w787, w786) -> (w785:bool)
          n438 = global read "GVZeitenZyklen.vi" "Big Ben, Methodenzeit, Zykluszeit0, Zykluszeit1, Zykluszeit2A, Zykluszeit2B"() -> (w780:dbl[])
          n439 = Index Array(array=w780, index=3 ("Index")) -> (element=w769:dbl)
          n440 = Greater Or Equal?(x=w769, y=w778) -> (x >= y?=w777:bool)
          n441 = Greater Or Equal?(x=w769, y=w772) -> (x >= y?=w775:bool)
          n442 = And(x=w775, y=w774) -> (x .and. y?=w771:bool)
          n443 = And(x=w777, y=w776) -> (x .and. y?=w766:bool)
          n444 = Or(x=w766, y=w771) -> (x .or. y?=w770:bool)
          n445 = And(x=w782, y=w770) -> (x .and. y?=w781:bool)
          n446 = case shown="True" w781 {
            tunnel: w784 -> [w790 w791]
            tunnel: [w790 w795] -> w783
            tunnel: w768 -> [_ w794]
            tunnel: w767 -> [_ w793]
            tunnel: w766 -> [_ w792]
            frame False {
            }
            frame True {
              n447 = call "MSDateienSchicken12-15.vi"("MSNummer"=w791, "MSa?"=w792, "Dateipfad:fromcriordy"=w793, "Dateipfad:fromcriocmd"=w794) -> ()  [unwired: 1 in]
              n448 = Increment(x=w791) -> (x+1=w795:i32)
            }
          }
        }
      }
      n449 = Add Array Elements(numeric array=w282) -> (sum=w357:i32)
      n450 = Index Array(array=w282, index #1=0 ("Index"), index #2=1 ("Index")) -> (element #1=w368:i32, element #2=w366:i32)
      n451 = Split 1D Array(array=w347, index=w368) -> (first subarray=w372:dbl[], second subarray=w376:dbl[])
      n452 = Split 1D Array(array=w283, index=w368) -> (first subarray=w375:string[], second subarray=w377:string[])
      n453 = Split 1D Array(array=w346, index=w368) -> (first subarray=w365:string[], second subarray=w367:string[])
      n454 = Initialize Array(-1.0 ("Element"), w357) -> (w344:dbl[])
      n455 = Split 1D Array(array=w377, index=w366) -> (first subarray=w374:string[], second subarray=w373:string[])
      n456 = Split 1D Array(array=w376, index=w366) -> (first subarray=w371:dbl[], second subarray=w370:dbl[])
      n457 = Split 1D Array(array=w367, index=w366) -> (first subarray=w364:string[], second subarray=w363:string[])
      n458 = Bundle(w375, w374, w373, w372, w371, w370) -> (w369:T16)  [unwired: 1 in]
      n459 = Bundle(w365, w364, w363) -> (w362:cluster{string[], string[], string[]})  [unwired: 1 in]
      n460 = Initialize Array(0.0, 8 ("Dimension")) -> (w294:dbl[])
      n461 = Bundle(w361, w361, w361) -> (w360:cluster{i32, i32, i32})  [unwired: 1 in]
      n462 = Initialize Array("x", 8 ("Dimension")) -> (w299:string[])
      n463 = case shown="True" TRUE ("SerielleKomm.") {
        tunnel: bool[] [TRUE, TRUE, TRUE, TRUE, TRUE, TRUE, TRUE, TRUE] -> [_ w430]
        tunnel: w299 -> [_ w429]
        tunnel: w369 -> [_ w428]
        tunnel: w368 -> [_ w427]
        tunnel: w366 -> [_ w426]
        tunnel: w362 -> [_ w425]
        tunnel: w360 -> [_ w424]
        tunnel: w359 -> [_ w423]
        tunnel: w347 -> [_ w422]
        tunnel: w345 -> [_ w421]
        tunnel: w344 -> [_ w420]
        tunnel: w343 -> [_ w417]
        tunnel: w322 -> [_ w419]
        tunnel: w294 -> [_ w418]
        tunnel: w293 -> [_ w416]
        frame False {
        }
        frame True {
          n464 = while {
            tunnel: w417 -> [w444]
            tunnel: w416 -> [w443]
            shift-right: [w442] -> _
            shift-left: errorcluster {"status"=FALSE, "code"=0, "source"=""} ("error out") -> [w441]
            stop <- w445 stop-if-true
            n465 = call "Warten6"("Count(mSec)"=u32 500) -> ()  [unwired: 1 out]
            n466 = global read "gvbooleschRT.vi" "global stop RT"() -> (w445:bool)
            n467 = case shown="True" "NeuerRefstrom" {
              tunnel: w443 -> [w447 _]
              tunnel: [w446 w456] -> w436
              tunnel: [w446 w459] -> w432
              frame False {
                n468 = String To Byte Array(string=w447) -> (unsigned byte array=w446:u8[])
              }
              frame True {
                n469 = local write "NeuerRefstrom"(FALSE ("NeuerRefstrom")) -> ()
                n470 = Number To Decimal String(number="RefStromECD1", width (-)=i16 4) -> (decimal integer string=w451:string)
                n471 = Number To Decimal String(number="RefStromECD2", width (-)=i16 4) -> (decimal integer string=w448:string)
                n472 = Concatenate Strings("?SE0,SETP," ("string"), w451, "\n") -> (w460:string)
                n473 = Concatenate Strings("?SE0,SETP," ("string"), w448, "\n") -> (w457:string)
                n474 = String To Byte Array(string=w460) -> (unsigned byte array=w459:u8[])
                n475 = String To Byte Array(string=w457) -> (unsigned byte array=w456:u8[])
              }
            }
            n476 = Join Numbers(hi=w432, lo=u8 5) -> ((hi.lo)=w438:u16[])
            n477 = Join Numbers(hi=w436, lo=u8 6) -> ((hi.lo)=w434:u16[])
            n478 = xnode "Invoke Method"("FPGA-VI-Referenz (Eingang)"=w444, "Fehler (Eingang)"=w441, "Daten"=w438) -> ("FPGA-VI-Referenz (Ausgang)"=w437:refnum<k20>, "Fehler (Ausgang)"=w433:errorcluster)  [unwired: 1 in, 1 out]
            n479 = xnode "Invoke Method"("FPGA-VI-Referenz (Eingang)"=w437, "Fehler (Eingang)"=w433, "Daten"=w434) -> ("Fehler (Ausgang)"=w442:errorcluster)  [unwired: 1 in, 2 out]
            "FIFOwriteRS485" <- w442
          }
          n480 = while {
            shift-right: [w470] -> _
            shift-left: w430 -> [w465]
            shift-right: [w484] -> _
            shift-left: w420 -> [w490]
            tunnel: w417 -> [w469]
            shift-right: [w471] -> _
            shift-left: w429 -> [w475]
            tunnel: w421 -> [w477]
            tunnel: w422 -> [w473]
            shift-right: [w478] -> _
            shift-left: w423 -> [w486]
            tunnel: w427 -> [w488]
            tunnel: w426 -> [w489]
            tunnel: w428 -> [w491]
            tunnel: w425 -> [w482]
            shift-right: [w479] -> _
            shift-left: w424 -> [w481]
            shift-right: [w467] -> _
            shift-left: w419 -> [w467]
            shift-right: [w464] -> _
            shift-left: w418 -> [w466]
            shift-right: [w472] -> _
            shift-left: errorcluster {"status"=FALSE, "code"=0, "source"=""} ("error out") -> [w468]
            stop <- w485 stop-if-true
            n481 = global read "GVHorstSP.vi" "HorstSP"() -> (w484:dbl[])
            n482 = Not Equal?(x=w484, y=w490) -> (x != y?=w487:bool)
            n483 = for {
              tunnel: w465 -> [w493] mode=indexing
              tunnel: w466 -> [w492] mode=indexing
              tunnel: [w499] -> w464 mode=indexing
              tunnel: [w496] -> w463 mode=indexing
              n484 = global read "GVZeitenZyklen.vi" "Big Ben, Methodenzeit, Zykluszeit0, Zykluszeit1, Zykluszeit2A, Zykluszeit2B"() -> (w502:dbl[])
              n485 = Index Array(array=w502, index=0 ("Index")) -> (element=w500:dbl)
              n486 = Subtract(x=w500, y=w492) -> (x-y=w498:dbl)
              n487 = Greater?(x=w498, y=0.1) -> (0:w495:bool)
              n488 = Or(x=w493, y=w495) -> (x .or. y?=w494:bool)
              n489 = Select(t=w495, s=w495, f=w493) -> (s? t:f=w496:bool)
              n490 = Select(t=w500, s=w494, f=w492) -> (s? t:f=w499:dbl)
            }
            n491 = call "NeueSP.vi"("Anzahl2"=w489, "Anzahl1"=w488, "AlteSP"=w490, 7:"NeueSP"=w484, "BefehleCluster"=w486, 10:"NeueSP"=w487, "ClusterFest"=w491) -> ("BefehleCluster"=w480:T17)  [unwired: 4 in]
            n492 = call "Warten3"("Count(mSec)"=u32 1) -> ()  [unwired: 1 out]
            n493 = call "Senden_ECD.vi"("error in"=w468, "BefehlsCluster"=w480, "AbfragenCluster"=w482, "Abfragenr.Cluster"=w481, "Senden?"=w463, "FPGA-VI-Referenz"=w469) -> ("BefehlsCluster"=w478:T17, "error out"=w474:errorcluster, "Senden?"=w476:bool[], "Abfragenr.Cluster"=w479:cluster{i32, i32, i32})  [unwired: 1 in]
            n494 = call "SeriellRead_ECD.vi"("SkalierungsfaktorHorst"=w473, "VorwortHorst"=w477, "error in"=w474, "Zwischenspeicher"=w475, "Senden?"=w476, "FPGA-VI-Referenz"=w469) -> ("Senden?"=w470:bool[], "Zwischenspeicher"=w471:string[], "error out"=w472:errorcluster)  [unwired: 3 in]
            "SerielleKomm." <- w472
            n495 = global read "gvbooleschRT.vi" "global stop RT"() -> (w485:bool)
          }
        }
      }
    }
    frame #2 {
      n496 = xnode "Element lesen/schreiben"("FPGA-VI-Referenz (Eingang)"=w1070, "global stop"=TRUE) -> ("FPGA-VI-Referenz (Ausgang)"=w1069:refnum<k20>)  [unwired: 1 in, 1 out]
      n497 = xnode "Close FPGA VI Reference"("FPGA-VI-Referenz (Eingang)"=w1069) -> ()  [unwired: 1 in, 1 out]
    }
    frame #3 {
    }
    frame #4 {
    }
  }
